vi "Autonomous Independent.vi"() -> ()   [LabVIEW 2015]
doc: "This VI is called when autonomous begins, and will automatically be terminated when autonomous ends. You can carry out timed or sensor driven robot movement independently without needing to return to the caller."
uses:
  <vilib>/Rock Robotics/WPI/RobotDrive/WPI_RobotDriveDevRef.ctl
  <vilib>/Rock Robotics/WPI/MotorControl/WPI_MotorControlDeviceRef.ctl
  <vilib>/Rock Robotics/WPI/MotorControl/WPI_MotorControlType.ctl
  <vilib>/Rock Robotics/SystemInterfaces/DIO/FPGA_DIOPWMChannel.ctl
  <vilib>/Rock Robotics/WPI/PWM/WPI_PWMDeadband.ctl
  <vilib>/Rock Robotics/WPI/CAN/Jaguar/SubVIs/WPI_CANJaguar_ControlMode.ctl
  <vilib>/Rock Robotics/WPI/CAN/TalonSRX/WPI_CANTalonSRX_APIControlMode.ctl
  <vilib>/Rock Robotics/WPI/Encoder/WPI_EncoderDevRef.ctl
  <vilib>/Rock Robotics/SystemInterfaces/Encoder/FPGA_EncoderIdx.ctl
  <vilib>/Rock Robotics/SystemInterfaces/Counter/FPGA_CounterCtrSystemIndex.ctl
  <vilib>/Rock Robotics/WPI/Encoder/WPI_EncoderType.ctl
  <vilib>/Rock Robotics/WPI/Utilities/WPI_GetSetVariantRefNum.vi
  Robot Global Data.vi
panel:
  in  "stop?":bool
  out "Pot Position":dbl
  in  "Angle(degrees)":dbl
  out "End?":bool
  out "End?":bool
  in  "Gear Setting":bool=TRUE
  in  "Distance (in)":dbl
  in  "Auto Choice":T1(ring)=enum."Low Bar"
  # "Be sure to right-click and choose Data Operations>>Make Current Value default if you want to save the array values with the VI"
  # "Move Forward at Dist. Test"
  # "Move Arms Down/Up Test"
  # "Low"
  # "High"
  # "<<Turn Until Vision Test"
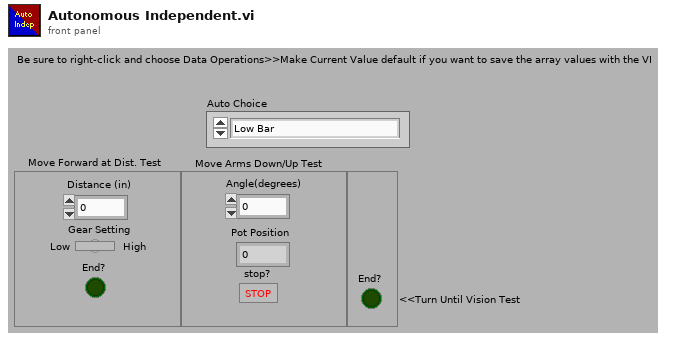
[diagram p1: front panel]
types:
  T1 = enum16{"Spybox/Shooting Test", "Low Bar", "Position 2", "Position 3", "Position 4", "Position 5", "Move Arms Down/Up Test", "Move Forward at Dist. Test", "Turn Until Vision Test"}
  T2 = typedef "WPI_RobotDriveDevRef.ctl" = cluster{"DevStatus":errorcluster, "Motors[]":T3[], "Square Inputs":bool, "Max Output":dbl}
  T3 = typedef "WPI_MotorControlDeviceRef.ctl" = cluster{"DeviceStatus":errorcluster, "Type":T4, "PWM":cluster{"PWM Channel":T5, "DeadBand":T6}, "CAN":cluster{"Device Number":u8, "Control Mode":T7, "Semaphore":T8, "Max Vout":dbl, "TalonSRX Control Mode":T9}, "Invert":bool}
  T4 = typedef "WPI_MotorControlType.ctl" = enum16{"PWM", "CAN", "CANTalonSRX"}
  T5 = typedef "FPGA_DIOPWMChannel.ctl" = enum8{"PWM 0", "PWM 1", "PWM 2", "PWM 3", "PWM 4", "PWM 5", "PWM 6", "PWM 7", "PWM 8", "PWM 9", "PWM MXP 0", "PWM MXP 1", "PWM MXP 2", "PWM MXP 3", "PWM MXP 4", "PWM MXP 5", "PWM MXP 6", "PWM MXP 7", "PWM MXP 8", "PWM MXP 9", "Invalid"}
  T6 = typedef "WPI_PWMDeadband.ctl" = cluster{"Name":string, "maxPositivePwm":i32, "minPositivePwm":i32, "centerPwm":i32, "maxNegativePwm":i32, "minNegativePwm":i32, "angularRange":u16}
  T7 = typedef "WPI_CANJaguar_ControlMode.ctl" = enum8{"Percent VBus", "Current", "Speed", "Position", "Voltage"}
  T8 = typedef "Semaphore RefNum" = refnum<k1>
  T9 = typedef "WPI_CANTalonSRX_APIControlMode.ctl" = enum8{"Percent VBus", "Speed", "Position", "Slave", "Unchanged / Invalid", "Voltage Compensation", "Current", "Motion Profile"}
  T10 = typedef "WPI_EncoderDevRef.ctl" = cluster{"DevStatus":errorcluster, "EncoderIndex":T11, "CounterIndex":T12, "DistancePerCount":dbl, "Decoding Type":T13}
  T11 = typedef "FPGA_EncoderIdx.ctl" = enum8{"Enc 0", "Enc 1", "Enc 2", "Enc 3", "Enc 4", "Enc 5", "Enc 6", "Enc 7", "Invalid"}
  T12 = typedef "FPGA_CounterCtrSystemIndex.ctl" = enum8{"Ctr 0", "Ctr 1", "Ctr 2", "Ctr 3", "Ctr 4", "Ctr 5", "Ctr 6", "Ctr 7", "Invalid"}
  T13 = typedef "WPI_EncoderType.ctl" = enum16{"1x", "2x", "4x"}
  T14 = cluster{"DriveRef":T2, "LeftEncRef":T10, "RightEncRef":T10}
  T15 = typedef "WPI_CANTalonSRX_GlobalStatus.ctl" = cluster{"Applied Throttle":dbl, "Module Enabled":bool, "CAN Error":errorcluster, "Closed Loop Error":dbl, "Forward Limit Switch Closed":bool, "Reverse Limit Switch Closed":bool, "Sensor Position":dbl, "Sensor Velocity":dbl, "Current":dbl, "Sticky Fault - Over Temp":bool, "Sticky Fault - Under Voltage":bool, "Sticky Fault - Forward Limit":bool, "Sticky Fault - Reverse Limit":bool, "Sticky Fault - Forward Soft Limit":bool, "Sticky Fault - Reverse Soft Limit":bool, "Brake is Enabled":bool, "Encoder Position":dbl, "Encoder Velocity":dbl, "Encoder Index Count":dbl, "Encoder A Pin State":bool, "Encoder B Pin State":bool, "Encoder Index Pin State":bool, "Analog In":dbl, "Analog In Velocity":dbl, "Temperature (C)":dbl, "Battery Voltage":dbl, "Control 5 Is Supported":bool, "Current Profile Slot Select":dbl, "Pos Div 8":bool, "Vel Div 4":bool, "Pulse Width Position":i32, "Pulse Width Velocity":i32, "Pulse Width Rise To Rise (us)":i32, "Pulse Width Rise To Fall (us)":i32, "Mot Prof Active Is Under Run":bool, "Mot Prof Active Has Under Run":bool, "Mot Prof Active Is Last":bool, "Mot Prof Active Velocity Only":bool, "Mot Prof Active Is Valid":bool, "Mot Prof Buffer Is Full":bool, "Mot Prof Active Profile Slot Select":i32, "Mot Prof NextID":i32, "Mot Prof Count":i32, "Mot Prof Active Velocity":dbl, "Mot Prof Active Position":dbl, "Mot Prof Output Enable":i32}
  T16 = enum16{"Start", "Turn (No Vision)", "Turn (Vision)", "Shoot", "Turn Back", "Move Back", "End"}
  T17 = cluster{"Angle":dbl, "Distance":dbl, "x":dbl, "y":dbl}
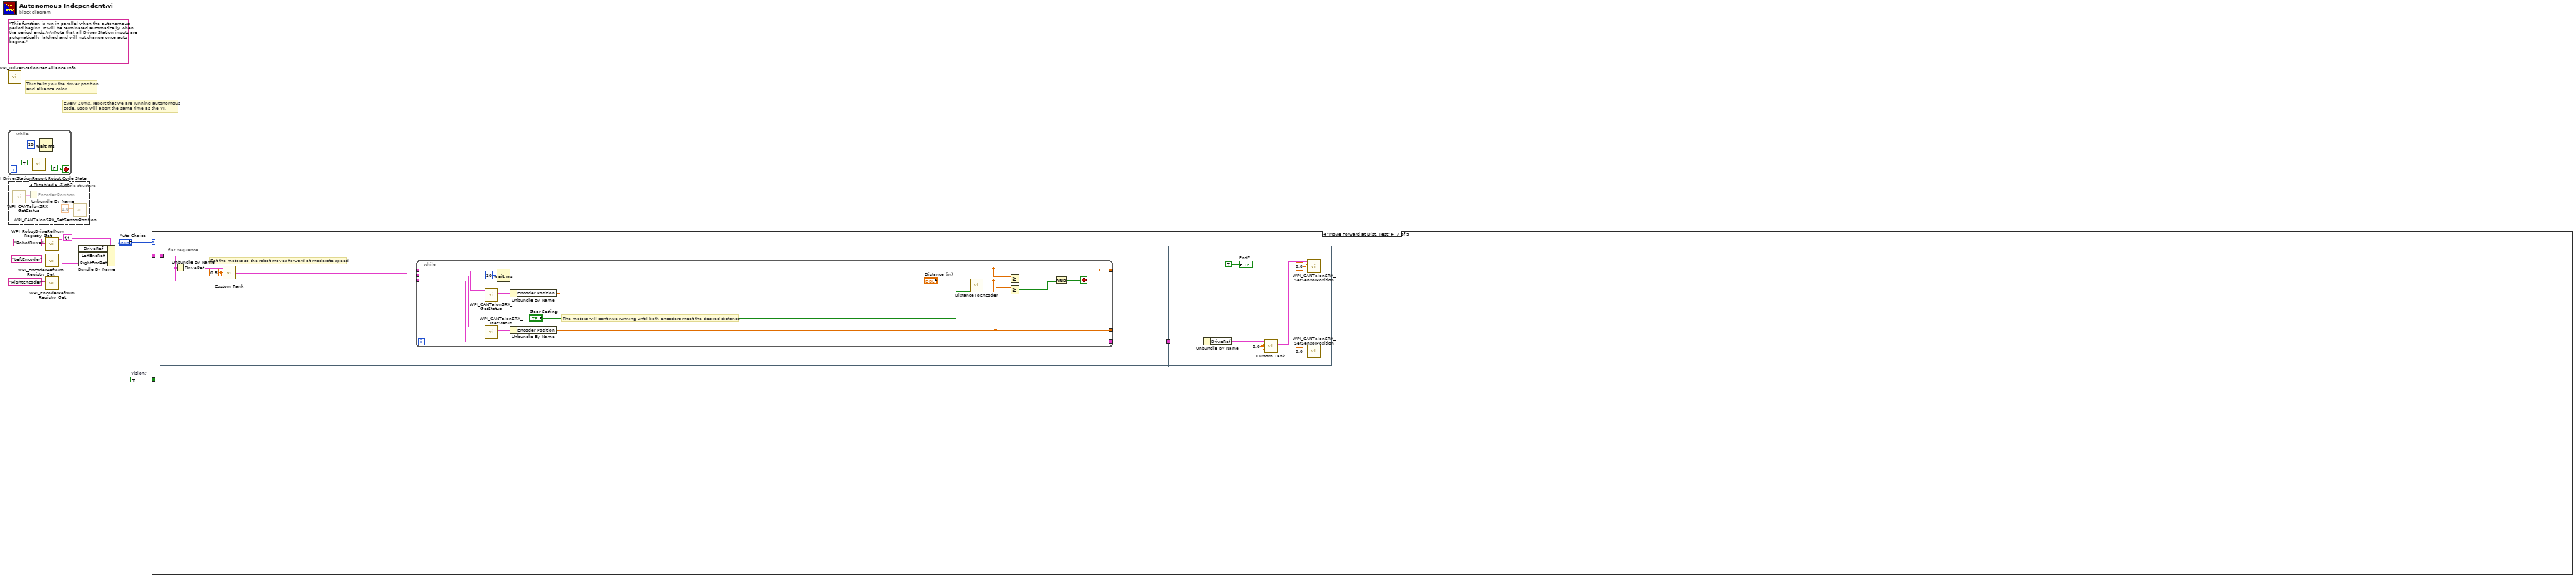
[diagram p0: block diagram]
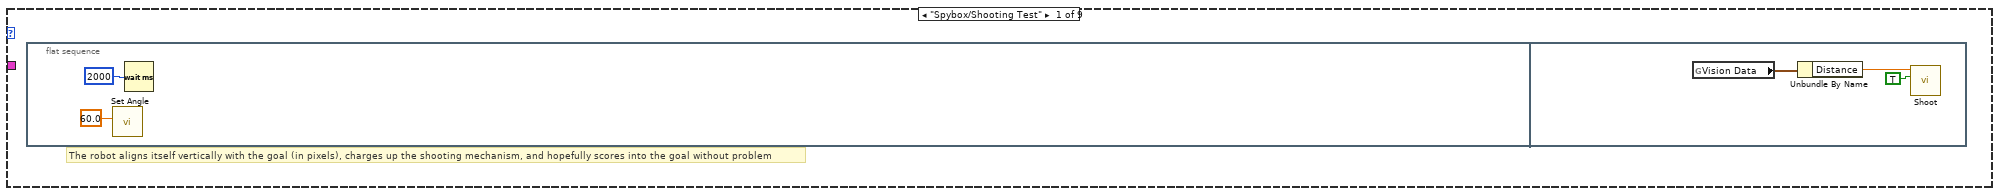
[diagram p3: hidden frame]
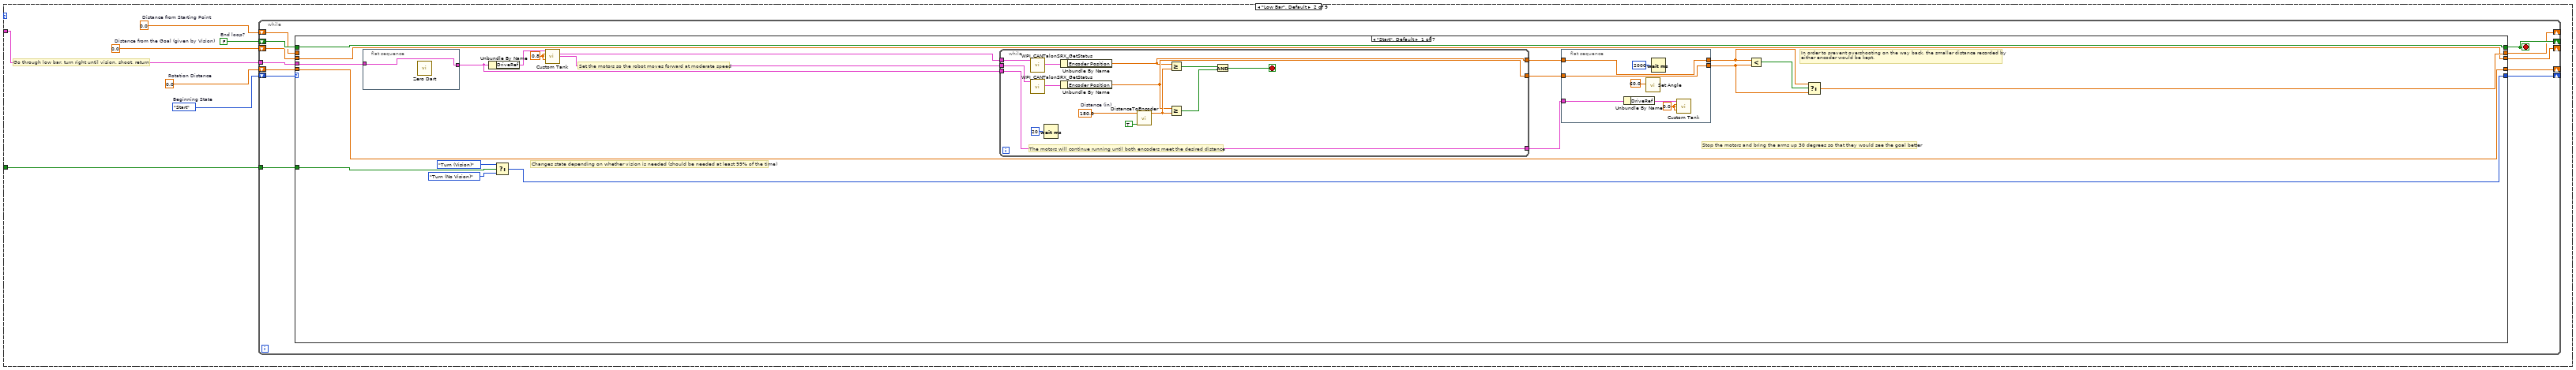
[diagram p4: hidden frame]
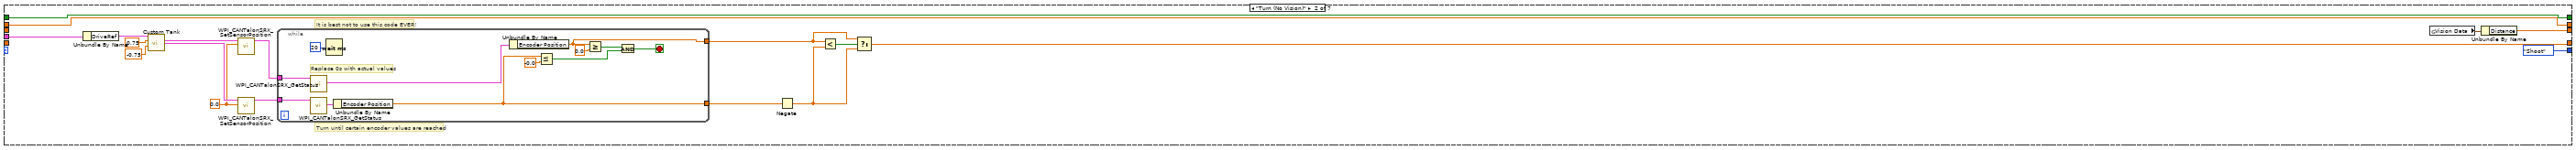
[diagram p5: hidden frame]
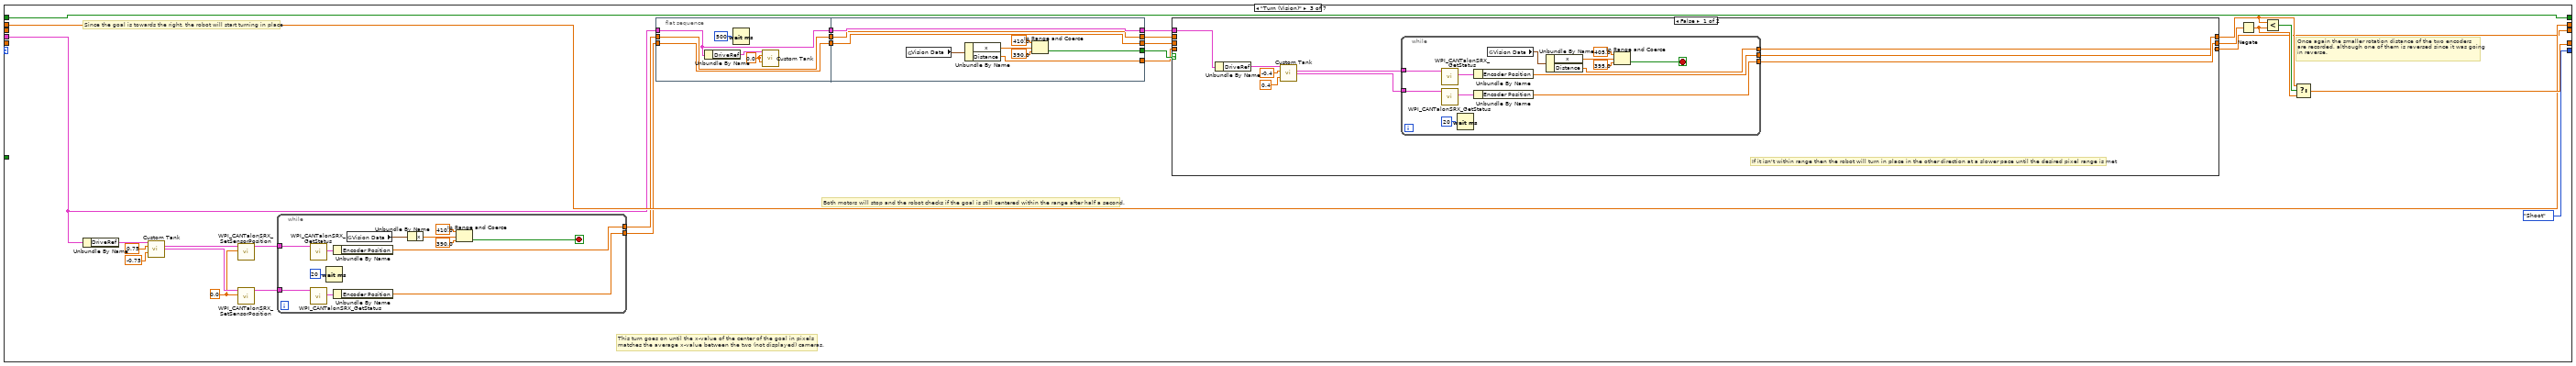
[diagram p6: hidden frame]
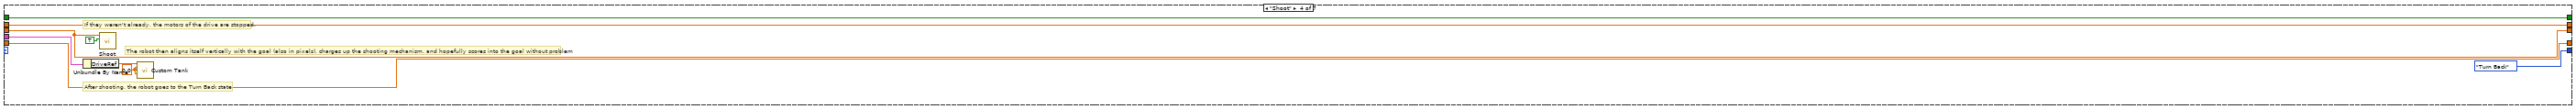
[diagram p8: hidden frame]
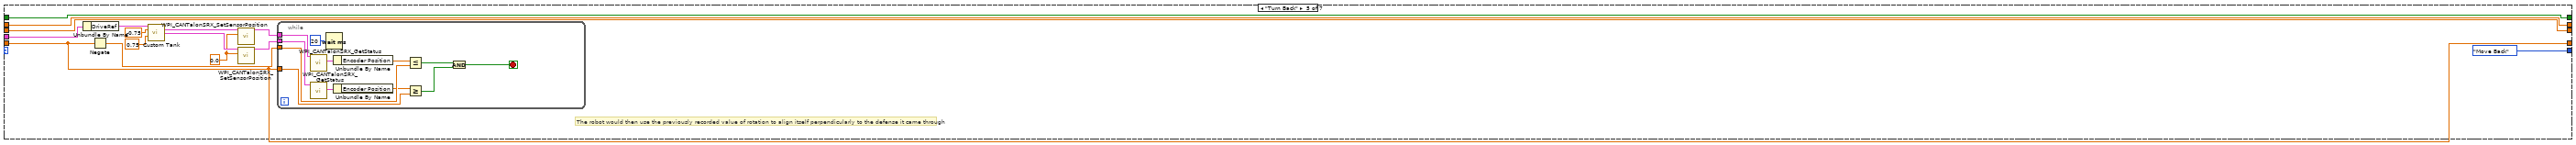
[diagram p9: hidden frame]
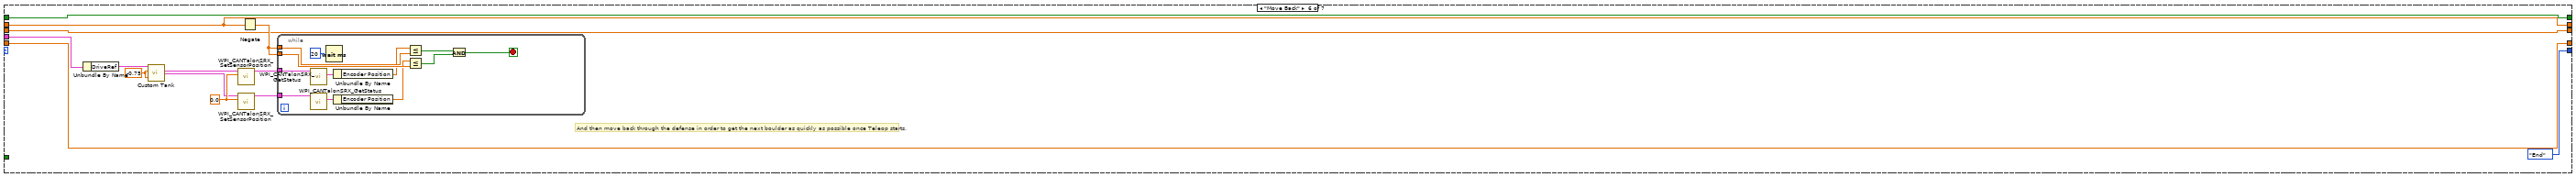
[diagram p10: hidden frame]
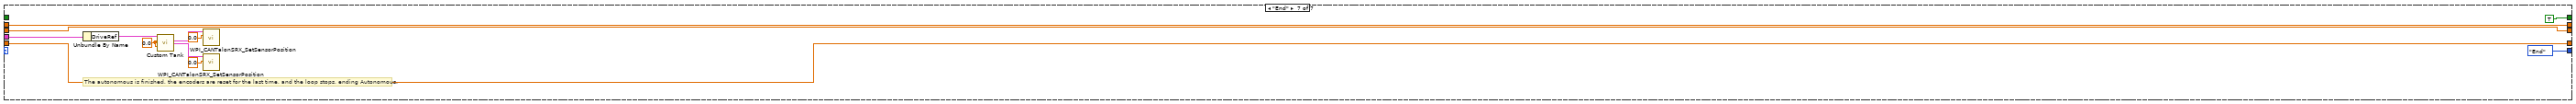
[diagram p11: hidden frame]
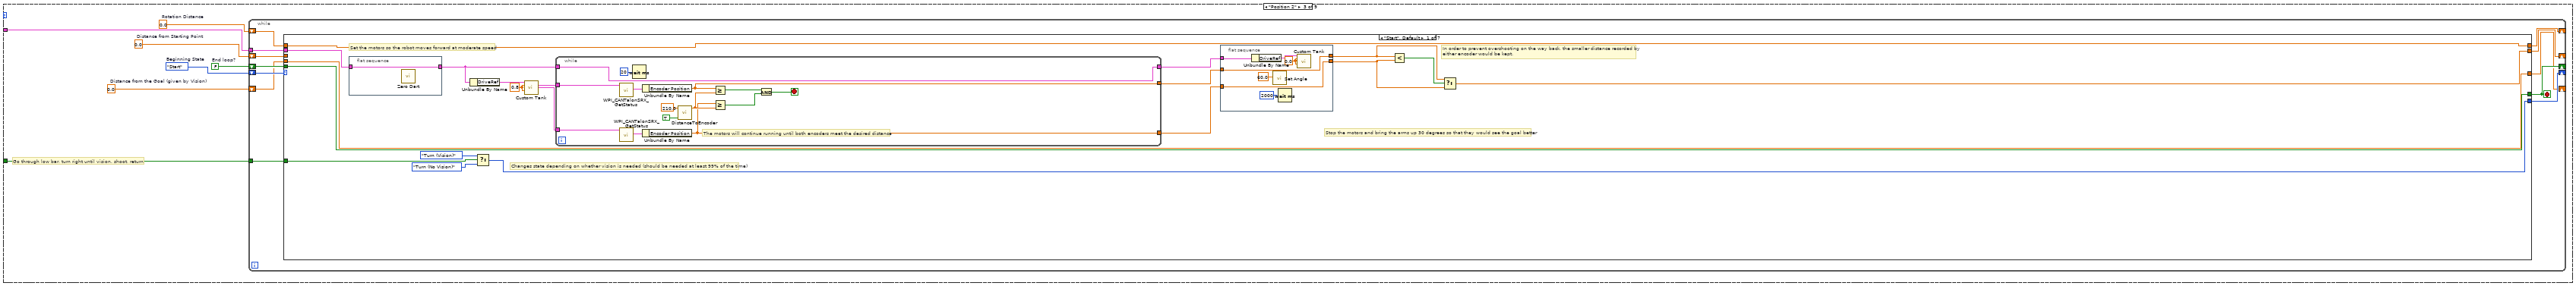
[diagram p12: hidden frame]
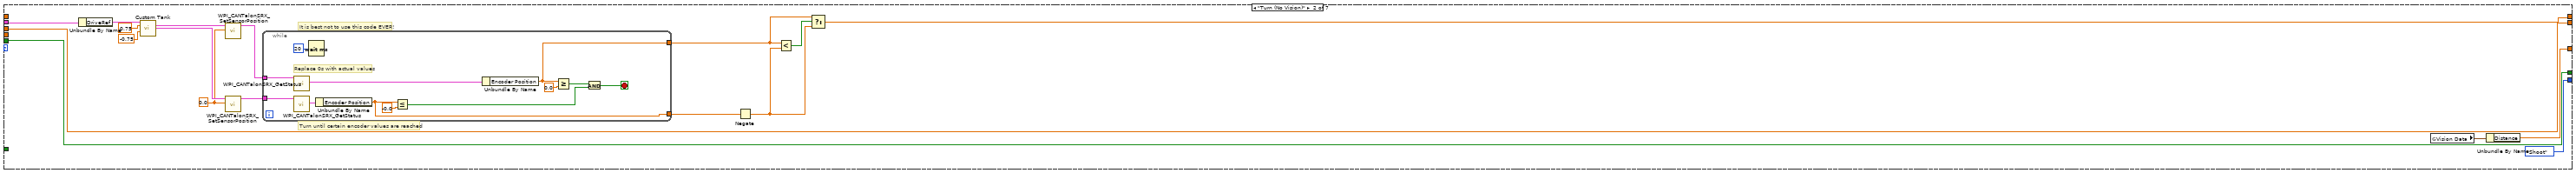
[diagram p13: hidden frame]
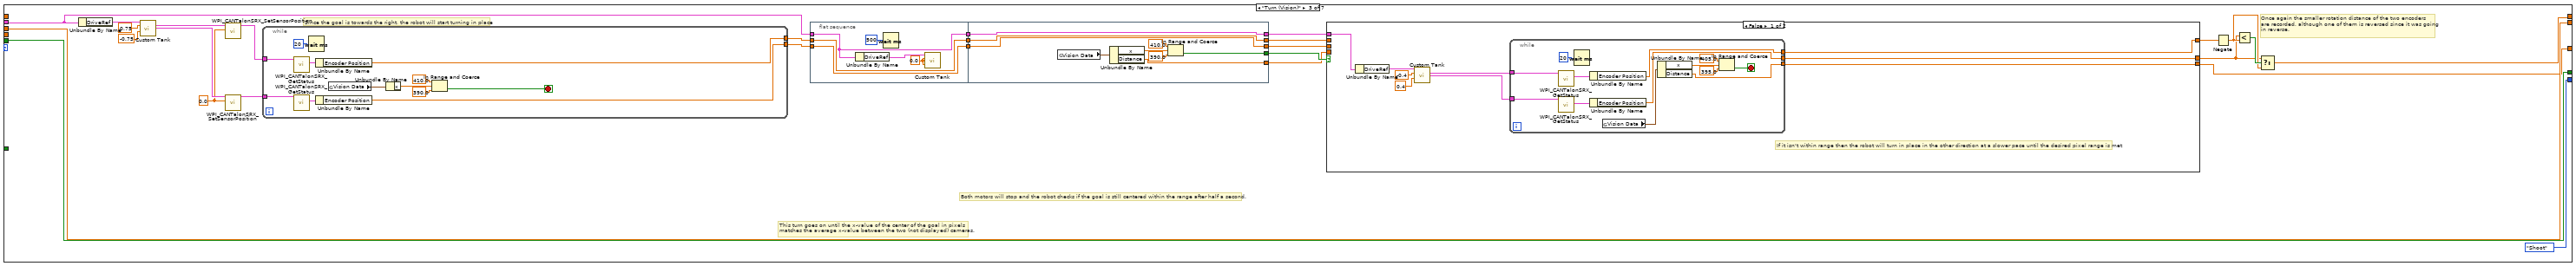
[diagram p14: hidden frame]
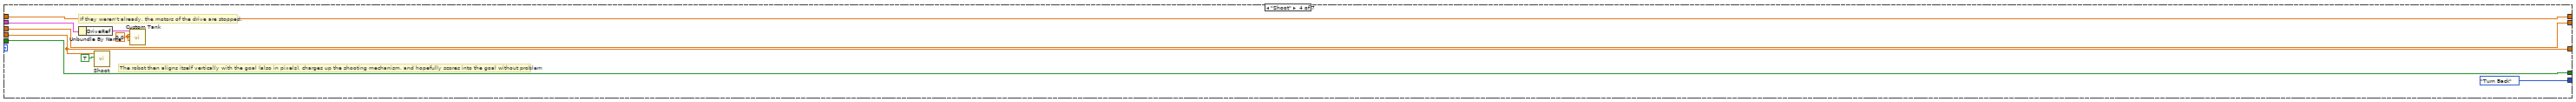
[diagram p16: hidden frame]
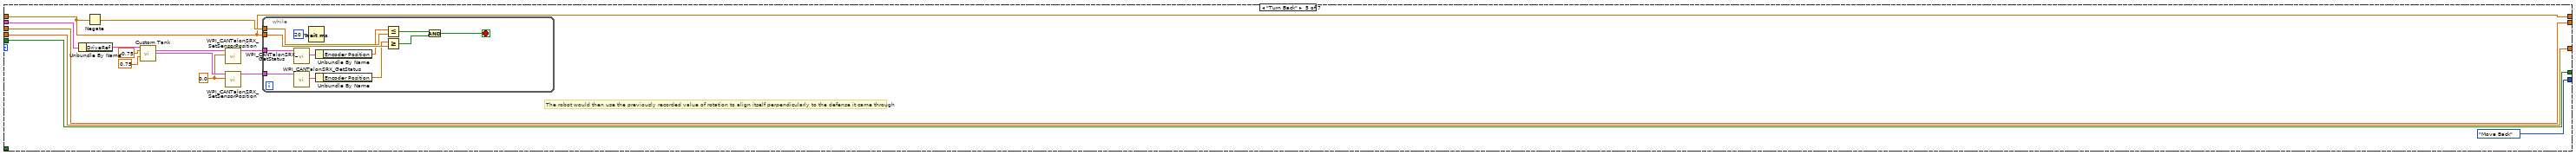
[diagram p17: hidden frame]
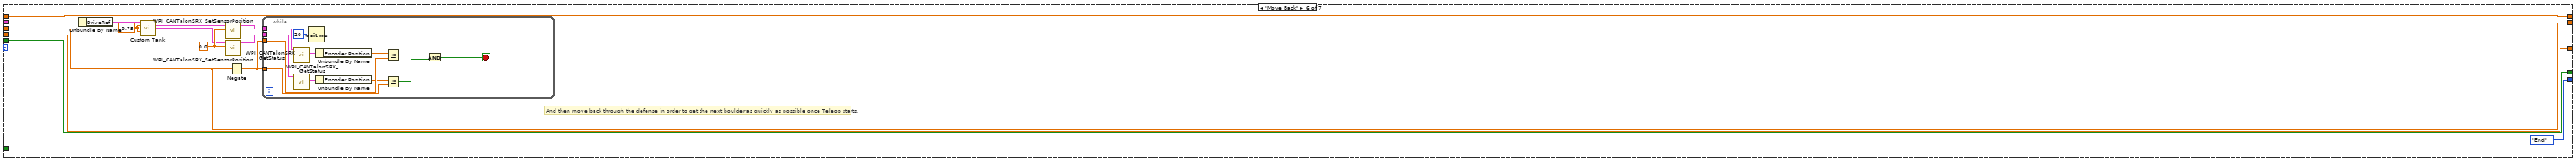
[diagram p18: hidden frame]
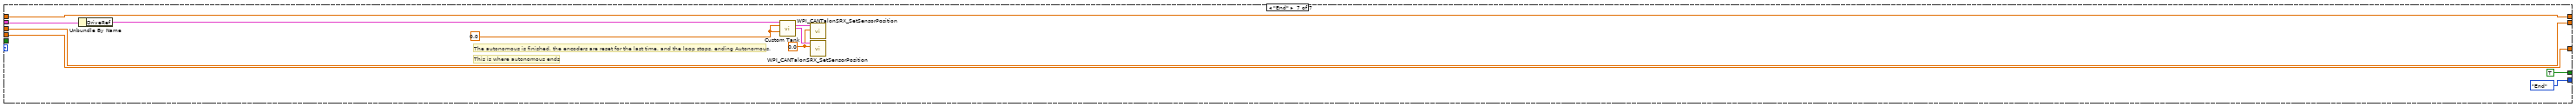
[diagram p19: hidden frame]
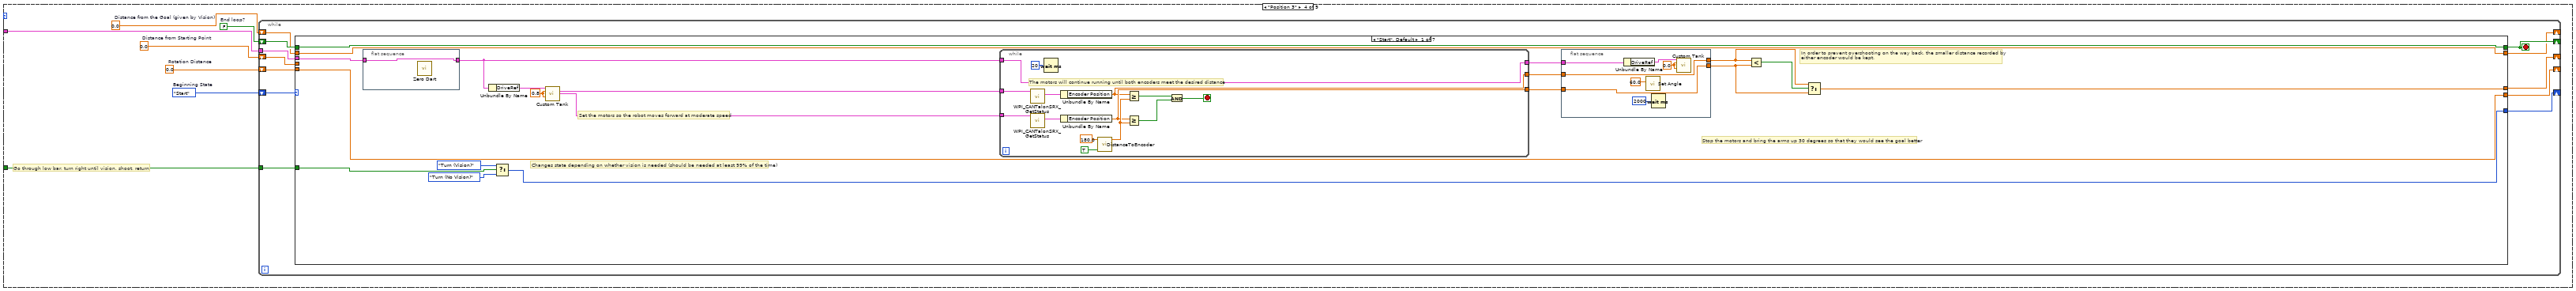
[diagram p20: hidden frame]
diagram:
  w10 = TRUE  # Vision?
  (unwired) "This function is run in parallel when the autonomous period begins. It will be terminated automatically when the period ends.\n\nNote that all Driver Station inputs are automatically latched and will not change once auto begins."
  # "Every 20ms, report that we are running autonomous\ncode. Loop will abort the same time as the VI."
  # "This tells you the driver position\nand alliance color"
  n1 = call <vilib>:"WPI_DriverStationGet Alliance Info.vi"() -> ()  [unwired: 12 out]
  n2 = while {
    stop <- FALSE stop-if-true
    n3 = call <vilib>:"WPI_DriverStationReport Robot Code State.vi"("Autonomous"=TRUE) -> ()  [unwired: 10 in, 1 out]
    n4 = Wait (ms)(milliseconds to wait=u32 20) -> ()  [unwired: 1 out]
  }
  n5 = disable-structure shown="Disabled" {
    frame Disabled {
      n6 = call <vilib>:"WPI_CANTalonSRX_GetStatus.vi"() -> ("Talon SRX Status"=w15:T15)  [unwired: 9 in, 2 out]
      n7 = Unbundle By Name(w15) -> ()  [unwired: 1 out]
      n8 = call <vilib>:"WPI_CANTalonSRX_SetSensorPosition.vi"("New Sensor Position"=0.0) -> ()  [unwired: 9 in, 2 out]
    }
    frame Enabled {
    }
  }
  n9 = call <vilib>:"WPI_RobotDriveRefNum Registry Get.vi"("refnum name"="RobotDrive") -> ("RobotDriveDevRef"=w5:T2)  [unwired: 9 in, 1 out]
  n10 = call <vilib>:"WPI_EncoderRefNum Registry Get.vi"("refnum name"="LeftEncoder") -> ("EncoderDevRef"=w4:T10)  [unwired: 9 in, 1 out]
  n11 = call <vilib>:"WPI_EncoderRefNum Registry Get.vi"("refnum name"="RightEncoder") -> ("EncoderDevRef"=w3:T10)  [unwired: 9 in, 1 out]
  n12 = Bundle By Name(cluster=T14 {"DriveRef"={"DevStatus"={"status"=FALSE, "code"=0, "source"=""}, "Motors[]"=[], "Square Inputs"=FALSE, "Max Output"=1.0}, "LeftEncRef"={"DevStatus"={"status"=FALSE, "code"=0, "source"=""}, "EncoderIndex"=enum."Invalid", "CounterIndex"=enum."Invalid", "DistancePerCount"=1.0, "Decoding Type"=enum."4x"}, "RightEncRef"={"DevStatus"={"status"=FALSE, "code"=0, "source"=""}, "EncoderIndex"=enum."Invalid", "CounterIndex"=enum."Invalid", "DistancePerCount"=1.0, "Decoding Type"=enum."4x"}}, "DriveRef"=w5, "LeftEncRef"=w4, "RightEncRef"=w3) -> (w2:T14)
  n13 = case shown="\"Move Forward at Dist. Test\"" "Auto Choice" {
    tunnel: w10 -> [_ w24 w268 w513 _ w869 _ _ _]
    tunnel: w2 -> [_ w21 w267 w512 w762 w868 w1120 w1151 _]
    frame "Spybox/Shooting Test" {
      # "The robot aligns itself vertically with the goal (in pixels), charges up the shooting mechanism, and hopefully scores into the goal without problem"
      n14 = flat-sequence {
        frame #0 {
          n15 = call "Set Angle.vi"("Angle(degrees)"=60.0) -> ()  [unwired: 7 in, 4 out]
          n16 = Wait (ms)(milliseconds to wait=u32 2000) -> ()  [unwired: 1 out]
        }
        frame #1 {
          n17 = global read "Robot Global Data.vi" "Vision Data"() -> (w18:T17)
          n18 = Unbundle By Name(w18) -> ("Distance"=w20:dbl)
          n19 = call "Shoot.vi"("Trigger"=TRUE ("Aimbot?"), "Vision Distance"=w20) -> ()  [unwired: 7 in, 3 out]
        }
      }
    }
    frame "Low Bar", Default {
      w27 = 0.0  # Distance from the Goal (given by Vision)
      w23 = 0.0  # Rotation Distance
      w22 = 0.0  # Distance from Starting Point
      w25 = FALSE  # End loop?
      w26 = T16."Start"  # Beginning State
      # "Go through low bar, turn right until vision, shoot, return"
      n20 = while {
        shift-right: [w39] -> _
        shift-left: w26 -> [w29]
        shift-right: [w37] -> _
        shift-left: w25 -> [w38]
        shift-right: [w35] -> _
        shift-left: w22 -> [w36]
        shift-right: [w33] -> _
        shift-left: w23 -> [w34]
        shift-right: [w31] -> _
        shift-left: w27 -> [w32]
        tunnel: w24 -> [w30]
        tunnel: w21 -> [w28]
        stop <- w37 stop-if-true
        n21 = case shown="\"Start\", Default" w29 {
          tunnel: [w59 T16."Shoot" T16."Shoot" T16."Turn Back" T16."Move Back" T16."End" T16."End"] -> w39
          tunnel: [w58 w99 w136 w201 w215 w241 TRUE] -> w37
          tunnel: w38 -> [w58 w99 w136 w201 w215 w241 _]
          tunnel: [w52 w98 w135 w196 w214 w238 w264] -> w35
          tunnel: w36 -> [_ w98 w135 w196 w214 w238 w264]
          tunnel: w34 -> [w51 _ _ w199 w212 w240 w263]
          tunnel: [w51 w93 w137 w199 w212 w240 w263] -> w33
          tunnel: w32 -> [w46 _ _ w195 w211 w237 w262]
          tunnel: [w46 w91 w122 w195 w211 w237 w262] -> w31
          tunnel: w30 -> [w50 _ _ _ _ _ _]
          tunnel: w28 -> [w45 w90 w134 w198 w210 w236 w261]
          frame "Start", Default {
            w42 = 0.8 ("LeftMotorsSpeed")
            # "In order to prevent overshooting on the way back, the smaller distance recorded by\neither encoder would be kept."
            # "Stop the motors and bring the arms up 30 degrees so that they would see the goal better"
            # "Set the motors so the robot moves forward at moderate speed"
            # "Changes state depending on whether vision is needed (should be needed at least 99% of the time)"
            n22 = flat-sequence {
              tunnel: w45 -> [w60]
              tunnel: [w60] -> w44
              frame #0 {
                n23 = call "Zero Dart.vi"() -> ()  [unwired: 10 in, 2 out]
              }
            }
            n24 = Unbundle By Name(w44) -> ("DriveRef"=w43:T2)
            n25 = Select(t=T16."Turn (Vision)", s=w50, f=T16."Turn (No Vision)") -> (s? t:f=w59:T16)
            n26 = call "Custom Tank.vi"("RobotDriveDevRef 2"=w43, "Left axis value"=w42, "Right axis value"=w42) -> ("Middle Left Motor"=w41:T3, "Middle Right Motor"=w40:T3)  [unwired: 8 in, 3 out]
            n27 = while {
              tunnel: [w61] -> w48
              tunnel: [w62] -> w47
              tunnel: w44 -> [w67]
              tunnel: [w67] -> w49
              tunnel: w41 -> [w64]
              tunnel: w40 -> [w63]
              stop <- w72 stop-if-true
              w70 = 180.0  # Distance (in)
              # "The motors will continue running until both encoders meet the desired distance"
              n28 = call <vilib>:"WPI_CANTalonSRX_GetStatus.vi"("CAN Talon SRX Ref"=w64) -> ("Talon SRX Status"=w66:T15)  [unwired: 8 in, 2 out]
              n29 = call <vilib>:"WPI_CANTalonSRX_GetStatus.vi"("CAN Talon SRX Ref"=w63) -> ("Talon SRX Status"=w65:T15)  [unwired: 8 in, 2 out]
              n30 = Wait (ms)(milliseconds to wait=u32 20) -> ()  [unwired: 1 out]
              n31 = Unbundle By Name(w66) -> ("Encoder Position"=w61:dbl)
              n32 = Unbundle By Name(w65) -> ("Encoder Position"=w62:dbl)
              n33 = call "DistanceToEncoder.vi"("Gear Setting"=TRUE, "Distance (in)"=w70) -> ("Encoder Ticks"=w69:dbl)  [unwired: 9 in]
              n34 = Greater Or Equal?(x=w61, y=w69) -> (x >= y?=w74:bool)
              n35 = Greater Or Equal?(x=w62, y=w69) -> (x >= y?=w73:bool)
              n36 = And(x=w74, y=w73) -> (x .and. y?=w72:bool)
            }
            n37 = flat-sequence {
              tunnel: [w78] -> w54
              tunnel: [w77] -> w53
              tunnel: w49 -> [w79]
              tunnel: w48 -> [w78]
              tunnel: w47 -> [w77]
              frame #0 {
                w75 = 0.0 ("LeftMotorsSpeed")
                n38 = Unbundle By Name(w79) -> ("DriveRef"=w76:T2)
                n39 = call "Set Angle.vi"("Angle(degrees)"=60.0) -> ()  [unwired: 7 in, 4 out]
                n40 = Wait (ms)(milliseconds to wait=u32 2000) -> ()  [unwired: 1 out]
                n41 = call "Custom Tank.vi"("RobotDriveDevRef 2"=w76, "Left axis value"=w75, "Right axis value"=w75) -> ()  [unwired: 8 in, 5 out]
              }
            }
            n42 = Less?(x=w54, y=w53) -> (x < y?=w55:bool)
            n43 = Select(t=w54, s=w55, f=w53) -> (s? t:f=w52:dbl)
          }
          frame "Turn (No Vision)" {
            w82 = 0.0 ("New Sensor Position")
            # "It is best not to use this code EVER!"
            # "Turn until certain encoder values are reached"
            n44 = Unbundle By Name(w90) -> ("DriveRef"=w89:T2)
            n45 = call "Custom Tank.vi"("RobotDriveDevRef 2"=w89, "Left axis value"=0.75 ("LeftMotorsSpeed"), "Right axis value"=-0.75 ("RightMotorsSpeed")) -> ("Middle Left Motor"=w86:T3, "Middle Right Motor"=w85:T3)  [unwired: 8 in, 3 out]
            n46 = call <vilib>:"WPI_CANTalonSRX_SetSensorPosition.vi"("New Sensor Position"=w82, "CAN Talon SRX Ref"=w86) -> ("CAN Talon SRX Ref"=w84:T3)  [unwired: 8 in, 1 out]
            n47 = call <vilib>:"WPI_CANTalonSRX_SetSensorPosition.vi"("New Sensor Position"=w82, "CAN Talon SRX Ref"=w85) -> ("CAN Talon SRX Ref"=w83:T3)  [unwired: 8 in, 1 out]
            n48 = while {
              tunnel: w84 -> [w105]
              tunnel: w83 -> [w103]
              tunnel: [w101] -> w95
              tunnel: [w102] -> w97
              stop <- w108 stop-if-true
              # "Replace 0s with actual values"
              n49 = call <vilib>:"WPI_CANTalonSRX_GetStatus.vi"("CAN Talon SRX Ref"=w105) -> ("Talon SRX Status"=w106:T15)  [unwired: 8 in, 2 out]
              n50 = call <vilib>:"WPI_CANTalonSRX_GetStatus.vi"("CAN Talon SRX Ref"=w103) -> ("Talon SRX Status"=w104:T15)  [unwired: 8 in, 2 out]
              n51 = Wait (ms)(milliseconds to wait=u32 20) -> ()  [unwired: 1 out]
              n52 = Unbundle By Name(w104) -> ("Encoder Position"=w102:dbl)
              n53 = Unbundle By Name(w106) -> ("Encoder Position"=w101:dbl)
              n54 = Less Or Equal?(x=w102, y=-0.0) -> (x <= y?=w110:bool)
              n55 = Greater Or Equal?(x=w101, y=0.0) -> (x >= y?=w111:bool)
              n56 = And(x=w111, y=w110) -> (x .and. y?=w108:bool)
            }
            n57 = Negate(x=w97) -> (-x=w94:dbl)
            n58 = Less?(x=w95, y=w94) -> (x < y?=w96:bool)
            n59 = Select(t=w95, s=w96, f=w94) -> (s? t:f=w93:dbl)
            n60 = global read "Robot Global Data.vi" "Vision Data"() -> (w92:T17)
            n61 = Unbundle By Name(w92) -> ("Distance"=w91:dbl)
          }
          frame "Turn (Vision)" {
            w113 = 0.0 ("New Sensor Position")
            # "This turn goes on until the x-value of the center of the goal in pixels\nmatches the average x-value between the two (not displayed) cameras."
            # "Once again the smaller rotation distance of the two encoders\nare recorded, although one of them is reversed since it was going\nin reverse."
            # "Both motors will stop and the robot checks if the goal is still centered within the range after half a second."
            # "Since the goal is towards the right, the robot will start turning in place"
            n62 = Unbundle By Name(w134) -> ("DriveRef"=w120:T2)
            n63 = call "Custom Tank.vi"("RobotDriveDevRef 2"=w120, "Left axis value"=0.75 ("LeftMotorsSpeed"), "Right axis value"=-0.75 ("RightMotorsSpeed")) -> ("Middle Left Motor"=w117:T3, "Middle Right Motor"=w116:T3)  [unwired: 8 in, 3 out]
            n64 = call <vilib>:"WPI_CANTalonSRX_SetSensorPosition.vi"("New Sensor Position"=w113, "CAN Talon SRX Ref"=w117) -> ("CAN Talon SRX Ref"=w115:T3)  [unwired: 8 in, 1 out]
            n65 = call <vilib>:"WPI_CANTalonSRX_SetSensorPosition.vi"("New Sensor Position"=w113, "CAN Talon SRX Ref"=w116) -> ("CAN Talon SRX Ref"=w114:T3)  [unwired: 8 in, 1 out]
            n66 = while {
              tunnel: [w169] -> w132
              tunnel: [w168] -> w133
              tunnel: w115 -> [w167]
              tunnel: w114 -> [w166]
              stop <- w173 stop-if-true
              n67 = call <vilib>:"WPI_CANTalonSRX_GetStatus.vi"("CAN Talon SRX Ref"=w167) -> ("Talon SRX Status"=w171:T15)  [unwired: 8 in, 2 out]
              n68 = call <vilib>:"WPI_CANTalonSRX_GetStatus.vi"("CAN Talon SRX Ref"=w166) -> ("Talon SRX Status"=w170:T15)  [unwired: 8 in, 2 out]
              n69 = Wait (ms)(milliseconds to wait=u32 20) -> ()  [unwired: 1 out]
              n70 = Unbundle By Name(w171) -> ("Encoder Position"=w168:dbl)
              n71 = Unbundle By Name(w170) -> ("Encoder Position"=w169:dbl)
              n72 = global read "Robot Global Data.vi" "Vision Data"() -> (w177:T17)
              n73 = Unbundle By Name(w177) -> ("x"=w176:dbl)
              n74 = In Range and Coerce(upper limit=410.0, x=w176, lower limit=390.0) -> (In Range?=w173:bool)  [unwired: 1 out]
            }
            n75 = flat-sequence {
              tunnel: w134 -> [w182]
              tunnel: w133 -> [w181]
              tunnel: w132 -> [w180]
              tunnel: [w182] -> w126
              tunnel: [w181] -> w125
              tunnel: [w180] -> w124
              tunnel: [w190] -> w127
              tunnel: [w191] -> w128
              tunnel: [w192] -> w129
              tunnel: w126 -> [w192]
              tunnel: w125 -> [w191]
              tunnel: w124 -> [w190]
              tunnel: [w185] -> w123
              tunnel: [w184] -> w121
              frame #0 {
                w178 = 0.0 ("LeftMotorsSpeed")
                n76 = Unbundle By Name(w182) -> ("DriveRef"=w179:T2)
                n77 = Wait (ms)(milliseconds to wait=u32 500) -> ()  [unwired: 1 out]
                n78 = call "Custom Tank.vi"("RobotDriveDevRef 2"=w179, "Left axis value"=w178, "Right axis value"=w178) -> ()  [unwired: 8 in, 5 out]
              }
              frame #1 {
                n79 = global read "Robot Global Data.vi" "Vision Data"() -> (w189:T17)
                n80 = Unbundle By Name(w189) -> ("x"=w188:dbl, "Distance"=w184:dbl)
                n81 = In Range and Coerce(upper limit=410.0, x=w188, lower limit=390.0) -> (In Range?=w185:bool)  [unwired: 1 out]
              }
            }
            n82 = case shown="False" w123 {
              tunnel: [w148 w165] -> w130
              tunnel: w127 -> [_ w165]
              tunnel: w128 -> [_ w164]
              tunnel: [w149 w164] -> w131
              tunnel: w129 -> [w147 _]
              tunnel: [w146 w163] -> w122
              tunnel: w121 -> [_ w163]
              frame False {
                # "If it isn't within range then the robot will turn in place in the other direction at a slower pace until the desired pixel range is met"
                n83 = Unbundle By Name(w147) -> ("DriveRef"=w145:T2)
                n84 = call "Custom Tank.vi"("RobotDriveDevRef 2"=w145, "Left axis value"=-0.4 ("LeftMotorsSpeed"), "Right axis value"=0.4 ("RightMotorsSpeed")) -> ("Middle Left Motor"=w141:T3, "Middle Right Motor"=w142:T3)  [unwired: 8 in, 3 out]
                n85 = while {
                  tunnel: [w153] -> w149
                  tunnel: [w152] -> w148
                  tunnel: [w156] -> w146
                  tunnel: w142 -> [w151]
                  tunnel: w141 -> [w150]
                  stop <- w162 stop-if-true
                  n86 = call <vilib>:"WPI_CANTalonSRX_GetStatus.vi"("CAN Talon SRX Ref"=w150) -> ("Talon SRX Status"=w155:T15)  [unwired: 8 in, 2 out]
                  n87 = call <vilib>:"WPI_CANTalonSRX_GetStatus.vi"("CAN Talon SRX Ref"=w151) -> ("Talon SRX Status"=w154:T15)  [unwired: 8 in, 2 out]
                  n88 = Wait (ms)(milliseconds to wait=u32 20) -> ()  [unwired: 1 out]
                  n89 = Unbundle By Name(w155) -> ("Encoder Position"=w153:dbl)
                  n90 = Unbundle By Name(w154) -> ("Encoder Position"=w152:dbl)
                  n91 = global read "Robot Global Data.vi" "Vision Data"() -> (w161:T17)
                  n92 = Unbundle By Name(w161) -> ("x"=w160:dbl, "Distance"=w156:dbl)
                  n93 = In Range and Coerce(upper limit=405.0, x=w160, lower limit=395.0) -> (In Range?=w162:bool)  [unwired: 1 out]
                }
              }
              frame True {
                # "If it is within range, then the robot moves on to the shooting state"
              }
            }
            n94 = Negate(x=w130) -> (-x=w139:dbl)
            n95 = Less?(x=w131, y=w139) -> (x < y?=w140:bool)
            n96 = Select(t=w131, s=w140, f=w139) -> (s? t:f=w137:dbl)
          }
          frame "Shoot" {
            w193 = 0.0 ("LeftMotorsSpeed")
            # "After shooting, the robot goes to the Turn Back state"
            # "If they weren't already, the motors of the drive are stopped."
            # "The robot then aligns itself vertically with the goal (also in pixels), charges up the shooting mechanism, and hopefully scores into the goal without problem"
            n97 = Unbundle By Name(w198) -> ("DriveRef"=w194:T2)
            n98 = call "Shoot.vi"("Trigger"=TRUE ("Collection Trigger"), "Vision Distance"=w195) -> ()  [unwired: 7 in, 3 out]
            n99 = call "Custom Tank.vi"("RobotDriveDevRef 2"=w194, "Left axis value"=w193, "Right axis value"=w193) -> ()  [unwired: 8 in, 5 out]
          }
          frame "Turn Back" {
            w202 = 0.0 ("New Sensor Position")
            # "The robot would then use the previously recorded value of rotation to align itself perpendicularly to the defense it came through"
            n100 = Unbundle By Name(w210) -> ("DriveRef"=w209:T2)
            n101 = Negate(x=w212) -> (-x=w213:dbl)
            n102 = call "Custom Tank.vi"("RobotDriveDevRef 2"=w209, "Left axis value"=-0.75 ("LeftMotorsSpeed"), "Right axis value"=0.75 ("RightMotorsSpeed")) -> ("Middle Left Motor"=w203:T3, "Middle Right Motor"=w204:T3)  [unwired: 8 in, 3 out]
            n103 = call <vilib>:"WPI_CANTalonSRX_SetSensorPosition.vi"("New Sensor Position"=w202, "CAN Talon SRX Ref"=w203) -> ("CAN Talon SRX Ref"=w206:T3)  [unwired: 8 in, 1 out]
            n104 = call <vilib>:"WPI_CANTalonSRX_SetSensorPosition.vi"("New Sensor Position"=w202, "CAN Talon SRX Ref"=w204) -> ("CAN Talon SRX Ref"=w205:T3)  [unwired: 8 in, 1 out]
            n105 = while {
              tunnel: w206 -> [w218]
              tunnel: w205 -> [w217]
              tunnel: w212 -> [w225]
              tunnel: w213 -> [w224]
              stop <- w226 stop-if-true
              n106 = call <vilib>:"WPI_CANTalonSRX_GetStatus.vi"("CAN Talon SRX Ref"=w218) -> ("Talon SRX Status"=w222:T15)  [unwired: 8 in, 2 out]
              n107 = call <vilib>:"WPI_CANTalonSRX_GetStatus.vi"("CAN Talon SRX Ref"=w217) -> ("Talon SRX Status"=w221:T15)  [unwired: 8 in, 2 out]
              n108 = Wait (ms)(milliseconds to wait=u32 20) -> ()  [unwired: 1 out]
              n109 = Unbundle By Name(w222) -> ("Encoder Position"=w219:dbl)
              n110 = Unbundle By Name(w221) -> ("Encoder Position"=w220:dbl)
              n111 = Less Or Equal?(x=w219, y=w224) -> (x <= y?=w228:bool)
              n112 = Greater Or Equal?(x=w220, y=w225) -> (x >= y?=w227:bool)
              n113 = And(x=w228, y=w227) -> (x .and. y?=w226:bool)
            }
          }
          frame "Move Back" {
            w233 = 0.0 ("New Sensor Position")
            w234 = -0.75 ("LeftMotorsSpeed")
            # "And then move back through the defense in order to get the next boulder as quickly as possible once Teleop starts."
            n114 = Unbundle By Name(w236) -> ("DriveRef"=w235:T2)
            n115 = call "Custom Tank.vi"("RobotDriveDevRef 2"=w235, "Left axis value"=w234, "Right axis value"=w234) -> ("Middle Left Motor"=w232:T3, "Middle Right Motor"=w231:T3)  [unwired: 8 in, 3 out]
            n116 = call <vilib>:"WPI_CANTalonSRX_SetSensorPosition.vi"("New Sensor Position"=w233, "CAN Talon SRX Ref"=w232) -> ("CAN Talon SRX Ref"=w230:T3)  [unwired: 8 in, 1 out]
            n117 = call <vilib>:"WPI_CANTalonSRX_SetSensorPosition.vi"("New Sensor Position"=w233, "CAN Talon SRX Ref"=w231) -> ("CAN Talon SRX Ref"=w229:T3)  [unwired: 8 in, 1 out]
            n118 = Negate(x=w238) -> (-x=w239:dbl)
            n119 = while {
              tunnel: w230 -> [w246]
              tunnel: w229 -> [w243]
              tunnel: w239 -> [w251]
              tunnel: w239 -> [w250]
              stop <- w252 stop-if-true
              n120 = call <vilib>:"WPI_CANTalonSRX_GetStatus.vi"("CAN Talon SRX Ref"=w246) -> ("Talon SRX Status"=w248:T15)  [unwired: 8 in, 2 out]
              n121 = call <vilib>:"WPI_CANTalonSRX_GetStatus.vi"("CAN Talon SRX Ref"=w243) -> ("Talon SRX Status"=w245:T15)  [unwired: 8 in, 2 out]
              n122 = Wait (ms)(milliseconds to wait=u32 20) -> ()  [unwired: 1 out]
              n123 = Unbundle By Name(w248) -> ("Encoder Position"=w247:dbl)
              n124 = Unbundle By Name(w245) -> ("Encoder Position"=w244:dbl)
              n125 = Less Or Equal?(x=w247, y=w251) -> (x <= y?=w254:bool)
              n126 = Less Or Equal?(x=w244, y=w250) -> (x <= y?=w253:bool)
              n127 = And(x=w254, y=w253) -> (x .and. y?=w252:bool)
            }
          }
          frame "End" {
            w259 = 0.0 ("Left axis value")
            # "The autonomous is finished, the encoders are reset for the last time, and the loop stops, ending Autonomous."
            n128 = Unbundle By Name(w261) -> ("DriveRef"=w260:T2)
            n129 = call "Custom Tank.vi"("RobotDriveDevRef 2"=w260, "Left axis value"=w259, "Right axis value"=w259) -> ("Middle Left Motor"=w256:T3, "Middle Right Motor"=w255:T3)  [unwired: 8 in, 3 out]
            n130 = call <vilib>:"WPI_CANTalonSRX_SetSensorPosition.vi"("New Sensor Position"=0.0, "CAN Talon SRX Ref"=w256) -> ()  [unwired: 8 in, 2 out]
            n131 = call <vilib>:"WPI_CANTalonSRX_SetSensorPosition.vi"("New Sensor Position"=0.0, "CAN Talon SRX Ref"=w255) -> ()  [unwired: 8 in, 2 out]
          }
        }
      }
    }
    frame "Position 2" {
      w269 = 0.0  # Distance from the Goal (given by Vision)
      w270 = 0.0  # Rotation Distance
      w271 = 0.0  # Distance from Starting Point
      w272 = FALSE  # End loop?
      w273 = T16."Start"  # Beginning State
      # "Go through low bar, turn right until vision, shoot, return"
      n132 = while {
        shift-right: [w284] -> _
        shift-left: w273 -> [w285]
        shift-right: [w282] -> _
        shift-left: w272 -> [w283]
        shift-right: [w280] -> _
        shift-left: w271 -> [w281]
        shift-right: [w278] -> _
        shift-left: w270 -> [w279]
        shift-right: [w276] -> _
        shift-left: w269 -> [w277]
        tunnel: w268 -> [w275]
        tunnel: w267 -> [w274]
        stop <- w282 stop-if-true
        n133 = case shown="\"Start\", Default" w285 {
          tunnel: [w305 T16."Shoot" T16."Shoot" T16."Turn Back" T16."Move Back" T16."End" T16."End"] -> w284
          tunnel: [w304 w345 w382 w447 w456 w487 TRUE] -> w282
          tunnel: w283 -> [w304 w345 w382 w447 w456 w487 _]
          tunnel: [w298 w344 w381 w445 w461 w484 w509] -> w280
          tunnel: w281 -> [_ w344 w381 w445 w461 w484 w509]
          tunnel: w279 -> [w297 _ _ w444 w459 w486 w508]
          tunnel: [w297 w339 w383 w444 w459 w486 w508] -> w278
          tunnel: w277 -> [w296 _ _ w441 w458 w483 w507]
          tunnel: [w296 w337 w368 w441 w458 w483 w507] -> w276
          tunnel: w275 -> [w295 _ _ _ _ _ _]
          tunnel: w274 -> [w288 w336 w378 w443 w457 w482 w506]
          frame "Start", Default {
            w290 = 0.8 ("LeftMotorsSpeed")
            # "In order to prevent overshooting on the way back, the smaller distance recorded by\neither encoder would be kept."
            # "Stop the motors and bring the arms up 30 degrees so that they would see the goal better"
            # "Set the motors so the robot moves forward at moderate speed"
            # "Changes state depending on whether vision is needed (should be needed at least 99% of the time)"
            n134 = flat-sequence {
              tunnel: w288 -> [w306]
              tunnel: [w306] -> w289
              frame #0 {
                n135 = call "Zero Dart.vi"() -> ()  [unwired: 10 in, 2 out]
              }
            }
            n136 = Unbundle By Name(w289) -> ("DriveRef"=w291:T2)
            n137 = Select(t=T16."Turn (Vision)", s=w295, f=T16."Turn (No Vision)") -> (s? t:f=w305:T16)
            n138 = call "Custom Tank.vi"("RobotDriveDevRef 2"=w291, "Left axis value"=w290, "Right axis value"=w290) -> ("Middle Left Motor"=w287:T3, "Middle Right Motor"=w286:T3)  [unwired: 8 in, 3 out]
            n139 = while {
              tunnel: [w311] -> w293
              tunnel: [w309] -> w292
              tunnel: w289 -> [w313]
              tunnel: [w313] -> w294
              tunnel: w287 -> [w308]
              tunnel: w286 -> [w307]
              stop <- w318 stop-if-true
              # "The motors will continue running until both encoders meet the desired distance"
              n140 = call <vilib>:"WPI_CANTalonSRX_GetStatus.vi"("CAN Talon SRX Ref"=w308) -> ("Talon SRX Status"=w312:T15)  [unwired: 8 in, 2 out]
              n141 = call <vilib>:"WPI_CANTalonSRX_GetStatus.vi"("CAN Talon SRX Ref"=w307) -> ("Talon SRX Status"=w310:T15)  [unwired: 8 in, 2 out]
              n142 = Wait (ms)(milliseconds to wait=u32 20) -> ()  [unwired: 1 out]
              n143 = Unbundle By Name(w312) -> ("Encoder Position"=w311:dbl)
              n144 = Unbundle By Name(w310) -> ("Encoder Position"=w309:dbl)
              n145 = call "DistanceToEncoder.vi"("Gear Setting"=TRUE, "Distance (in)"=210.0 ("Distance")) -> ("Encoder Ticks"=w316:dbl)  [unwired: 9 in]
              n146 = Greater Or Equal?(x=w311, y=w316) -> (x >= y?=w320:bool)
              n147 = Greater Or Equal?(x=w309, y=w316) -> (x >= y?=w319:bool)
              n148 = And(x=w320, y=w319) -> (x .and. y?=w318:bool)
            }
            n149 = flat-sequence {
              tunnel: [w324] -> w300
              tunnel: [w323] -> w299
              tunnel: w294 -> [w325]
              tunnel: w293 -> [w324]
              tunnel: w292 -> [w323]
              frame #0 {
                w321 = 0.0 ("LeftMotorsSpeed")
                n150 = Unbundle By Name(w325) -> ("DriveRef"=w322:T2)
                n151 = call "Set Angle.vi"("Angle(degrees)"=60.0) -> ()  [unwired: 7 in, 4 out]
                n152 = Wait (ms)(milliseconds to wait=u32 2000) -> ()  [unwired: 1 out]
                n153 = call "Custom Tank.vi"("RobotDriveDevRef 2"=w322, "Left axis value"=w321, "Right axis value"=w321) -> ()  [unwired: 8 in, 5 out]
              }
            }
            n154 = Less?(x=w300, y=w299) -> (x < y?=w301:bool)
            n155 = Select(t=w300, s=w301, f=w299) -> (s? t:f=w298:dbl)
          }
          frame "Turn (No Vision)" {
            w330 = 0.0 ("New Sensor Position")
            # "It is best not to use this code EVER!"
            # "Turn until certain encoder values are reached"
            n156 = Unbundle By Name(w336) -> ("DriveRef"=w335:T2)
            n157 = call "Custom Tank.vi"("RobotDriveDevRef 2"=w335, "Left axis value"=0.75 ("LeftMotorsSpeed"), "Right axis value"=-0.75 ("RightMotorsSpeed")) -> ("Middle Left Motor"=w332:T3, "Middle Right Motor"=w331:T3)  [unwired: 8 in, 3 out]
            n158 = call <vilib>:"WPI_CANTalonSRX_SetSensorPosition.vi"("New Sensor Position"=w330, "CAN Talon SRX Ref"=w332) -> ("CAN Talon SRX Ref"=w329:T3)  [unwired: 8 in, 1 out]
            n159 = call <vilib>:"WPI_CANTalonSRX_SetSensorPosition.vi"("New Sensor Position"=w330, "CAN Talon SRX Ref"=w331) -> ("CAN Talon SRX Ref"=w328:T3)  [unwired: 8 in, 1 out]
            n160 = while {
              tunnel: w329 -> [w352]
              tunnel: w328 -> [w349]
              tunnel: [w350] -> w341
              tunnel: [w347] -> w343
              stop <- w354 stop-if-true
              # "Replace 0s with actual values"
              n161 = call <vilib>:"WPI_CANTalonSRX_GetStatus.vi"("CAN Talon SRX Ref"=w352) -> ("Talon SRX Status"=w351:T15)  [unwired: 8 in, 2 out]
              n162 = call <vilib>:"WPI_CANTalonSRX_GetStatus.vi"("CAN Talon SRX Ref"=w349) -> ("Talon SRX Status"=w348:T15)  [unwired: 8 in, 2 out]
              n163 = Wait (ms)(milliseconds to wait=u32 20) -> ()  [unwired: 1 out]
              n164 = Unbundle By Name(w348) -> ("Encoder Position"=w347:dbl)
              n165 = Less Or Equal?(x=w347, y=-0.0) -> (x <= y?=w356:bool)
              n166 = Unbundle By Name(w351) -> ("Encoder Position"=w350:dbl)
              n167 = Greater Or Equal?(x=w350, y=0.0) -> (x >= y?=w357:bool)
              n168 = And(x=w357, y=w356) -> (x .and. y?=w354:bool)
            }
            n169 = Negate(x=w343) -> (-x=w340:dbl)
            n170 = Less?(x=w341, y=w340) -> (x < y?=w342:bool)
            n171 = Select(t=w341, s=w342, f=w340) -> (s? t:f=w339:dbl)
            n172 = global read "Robot Global Data.vi" "Vision Data"() -> (w338:T17)
            n173 = Unbundle By Name(w338) -> ("Distance"=w337:dbl)
          }
          frame "Turn (Vision)" {
            w361 = 0.0 ("New Sensor Position")
            # "This turn goes on until the x-value of the center of the goal in pixels\nmatches the average x-value between the two (not displayed) cameras."
            # "Once again the smaller rotation distance of the two encoders\nare recorded, although one of them is reversed since it was going\nin reverse."
            # "Both motors will stop and the robot checks if the goal is still centered within the range after half a second."
            # "Since the goal is towards the right, the robot will start turning in place"
            n174 = Unbundle By Name(w378) -> ("DriveRef"=w366:T2)
            n175 = call "Custom Tank.vi"("RobotDriveDevRef 2"=w366, "Left axis value"=0.75 ("LeftMotorsSpeed"), "Right axis value"=-0.75 ("RightMotorsSpeed")) -> ("Middle Left Motor"=w363:T3, "Middle Right Motor"=w362:T3)  [unwired: 8 in, 3 out]
            n176 = call <vilib>:"WPI_CANTalonSRX_SetSensorPosition.vi"("New Sensor Position"=w361, "CAN Talon SRX Ref"=w363) -> ("CAN Talon SRX Ref"=w360:T3)  [unwired: 8 in, 1 out]
            n177 = call <vilib>:"WPI_CANTalonSRX_SetSensorPosition.vi"("New Sensor Position"=w361, "CAN Talon SRX Ref"=w362) -> ("CAN Talon SRX Ref"=w359:T3)  [unwired: 8 in, 1 out]
            n178 = while {
              tunnel: w360 -> [w416]
              tunnel: w359 -> [w413]
              tunnel: [w415] -> w380
              tunnel: [w412] -> w379
              stop <- w419 stop-if-true
              n179 = call <vilib>:"WPI_CANTalonSRX_GetStatus.vi"("CAN Talon SRX Ref"=w416) -> ("Talon SRX Status"=w417:T15)  [unwired: 8 in, 2 out]
              n180 = call <vilib>:"WPI_CANTalonSRX_GetStatus.vi"("CAN Talon SRX Ref"=w413) -> ("Talon SRX Status"=w414:T15)  [unwired: 8 in, 2 out]
              n181 = Wait (ms)(milliseconds to wait=u32 20) -> ()  [unwired: 1 out]
              n182 = Unbundle By Name(w417) -> ("Encoder Position"=w415:dbl)
              n183 = Unbundle By Name(w414) -> ("Encoder Position"=w412:dbl)
              n184 = global read "Robot Global Data.vi" "Vision Data"() -> (w423:T17)
              n185 = Unbundle By Name(w423) -> ("x"=w422:dbl)
              n186 = In Range and Coerce(upper limit=410.0, x=w422, lower limit=390.0) -> (In Range?=w419:bool)  [unwired: 1 out]
            }
            n187 = flat-sequence {
              tunnel: w380 -> [w426]
              tunnel: w379 -> [w427]
              tunnel: w378 -> [w428]
              tunnel: [w428] -> w372
              tunnel: [w427] -> w371
              tunnel: [w426] -> w370
              tunnel: [w436] -> w375
              tunnel: [w437] -> w376
              tunnel: [w438] -> w377
              tunnel: w372 -> [w438]
              tunnel: w371 -> [w437]
              tunnel: w370 -> [w436]
              tunnel: [w431] -> w369
              tunnel: [w430] -> w367
              frame #0 {
                w425 = 0.0 ("LeftMotorsSpeed")
                n188 = Unbundle By Name(w428) -> ("DriveRef"=w424:T2)
                n189 = Wait (ms)(milliseconds to wait=u32 500) -> ()  [unwired: 1 out]
                n190 = call "Custom Tank.vi"("RobotDriveDevRef 2"=w424, "Left axis value"=w425, "Right axis value"=w425) -> ()  [unwired: 8 in, 5 out]
              }
              frame #1 {
                n191 = global read "Robot Global Data.vi" "Vision Data"() -> (w435:T17)
                n192 = Unbundle By Name(w435) -> ("x"=w434:dbl, "Distance"=w430:dbl)
                n193 = In Range and Coerce(upper limit=410.0, x=w434, lower limit=390.0) -> (In Range?=w431:bool)  [unwired: 1 out]
              }
            }
            n194 = case shown="False" w369 {
              tunnel: [w394 w411] -> w374
              tunnel: w375 -> [_ w411]
              tunnel: w376 -> [_ w410]
              tunnel: [w395 w410] -> w373
              tunnel: w377 -> [w393 _]
              tunnel: [w392 w409] -> w368
              tunnel: w367 -> [_ w409]
              frame False {
                # "If it isn't within range then the robot will turn in place in the other direction at a slower pace until the desired pixel range is met"
                n195 = Unbundle By Name(w393) -> ("DriveRef"=w391:T2)
                n196 = call "Custom Tank.vi"("RobotDriveDevRef 2"=w391, "Left axis value"=-0.4 ("LeftMotorsSpeed"), "Right axis value"=0.4 ("RightMotorsSpeed")) -> ("Middle Left Motor"=w388:T3, "Middle Right Motor"=w387:T3)  [unwired: 8 in, 3 out]
                n197 = while {
                  tunnel: [w398] -> w395
                  tunnel: [w400] -> w394
                  tunnel: [w402] -> w392
                  tunnel: w388 -> [w397]
                  tunnel: w387 -> [w396]
                  stop <- w408 stop-if-true
                  n198 = call <vilib>:"WPI_CANTalonSRX_GetStatus.vi"("CAN Talon SRX Ref"=w397) -> ("Talon SRX Status"=w401:T15)  [unwired: 8 in, 2 out]
                  n199 = call <vilib>:"WPI_CANTalonSRX_GetStatus.vi"("CAN Talon SRX Ref"=w396) -> ("Talon SRX Status"=w399:T15)  [unwired: 8 in, 2 out]
                  n200 = Wait (ms)(milliseconds to wait=u32 20) -> ()  [unwired: 1 out]
                  n201 = Unbundle By Name(w401) -> ("Encoder Position"=w400:dbl)
                  n202 = Unbundle By Name(w399) -> ("Encoder Position"=w398:dbl)
                  n203 = global read "Robot Global Data.vi" "Vision Data"() -> (w407:T17)
                  n204 = Unbundle By Name(w407) -> ("x"=w406:dbl, "Distance"=w402:dbl)
                  n205 = In Range and Coerce(upper limit=405.0, x=w406, lower limit=395.0) -> (In Range?=w408:bool)  [unwired: 1 out]
                }
              }
              frame True {
                # "If it is within range, then the robot moves on to the shooting state"
              }
            }
            n206 = Negate(x=w374) -> (-x=w385:dbl)
            n207 = Less?(x=w373, y=w385) -> (x < y?=w386:bool)
            n208 = Select(t=w373, s=w386, f=w385) -> (s? t:f=w383:dbl)
          }
          frame "Shoot" {
            w439 = 0.0 ("LeftMotorsSpeed")
            # "If they weren't already, the motors of the drive are stopped."
            # "The robot then aligns itself vertically with the goal (also in pixels), charges up the shooting mechanism, and hopefully scores into the goal without problem"
            n209 = Unbundle By Name(w443) -> ("DriveRef"=w440:T2)
            n210 = call "Shoot.vi"("Trigger"=TRUE ("Collection Trigger"), "Vision Distance"=w441) -> ()  [unwired: 7 in, 3 out]
            n211 = call "Custom Tank.vi"("RobotDriveDevRef 2"=w440, "Left axis value"=w439, "Right axis value"=w439) -> ()  [unwired: 8 in, 5 out]
          }
          frame "Turn Back" {
            w450 = 0.0 ("New Sensor Position")
            # "The robot would then use the previously recorded value of rotation to align itself perpendicularly to the defense it came through"
            n212 = Unbundle By Name(w457) -> ("DriveRef"=w455:T2)
            n213 = Negate(x=w459) -> (-x=w460:dbl)
            n214 = call "Custom Tank.vi"("RobotDriveDevRef 2"=w455, "Left axis value"=-0.75 ("LeftMotorsSpeed"), "Right axis value"=0.75 ("RightMotorsSpeed")) -> ("Middle Left Motor"=w452:T3, "Middle Right Motor"=w451:T3)  [unwired: 8 in, 3 out]
            n215 = call <vilib>:"WPI_CANTalonSRX_SetSensorPosition.vi"("New Sensor Position"=w450, "CAN Talon SRX Ref"=w452) -> ("CAN Talon SRX Ref"=w449:T3)  [unwired: 8 in, 1 out]
            n216 = call <vilib>:"WPI_CANTalonSRX_SetSensorPosition.vi"("New Sensor Position"=w450, "CAN Talon SRX Ref"=w451) -> ("CAN Talon SRX Ref"=w448:T3)  [unwired: 8 in, 1 out]
            n217 = while {
              tunnel: w449 -> [w466]
              tunnel: w448 -> [w463]
              tunnel: w459 -> [w471]
              tunnel: w460 -> [w470]
              stop <- w472 stop-if-true
              n218 = call <vilib>:"WPI_CANTalonSRX_GetStatus.vi"("CAN Talon SRX Ref"=w466) -> ("Talon SRX Status"=w468:T15)  [unwired: 8 in, 2 out]
              n219 = call <vilib>:"WPI_CANTalonSRX_GetStatus.vi"("CAN Talon SRX Ref"=w463) -> ("Talon SRX Status"=w465:T15)  [unwired: 8 in, 2 out]
              n220 = Wait (ms)(milliseconds to wait=u32 20) -> ()  [unwired: 1 out]
              n221 = Unbundle By Name(w468) -> ("Encoder Position"=w467:dbl)
              n222 = Unbundle By Name(w465) -> ("Encoder Position"=w464:dbl)
              n223 = Less Or Equal?(x=w467, y=w470) -> (x <= y?=w474:bool)
              n224 = Greater Or Equal?(x=w464, y=w471) -> (x >= y?=w473:bool)
              n225 = And(x=w474, y=w473) -> (x .and. y?=w472:bool)
            }
          }
          frame "Move Back" {
            w479 = 0.0 ("New Sensor Position")
            w480 = -0.75 ("LeftMotorsSpeed")
            # "And then move back through the defense in order to get the next boulder as quickly as possible once Teleop starts."
            n226 = Unbundle By Name(w482) -> ("DriveRef"=w481:T2)
            n227 = call "Custom Tank.vi"("RobotDriveDevRef 2"=w481, "Left axis value"=w480, "Right axis value"=w480) -> ("Middle Left Motor"=w478:T3, "Middle Right Motor"=w477:T3)  [unwired: 8 in, 3 out]
            n228 = call <vilib>:"WPI_CANTalonSRX_SetSensorPosition.vi"("New Sensor Position"=w479, "CAN Talon SRX Ref"=w478) -> ("CAN Talon SRX Ref"=w476:T3)  [unwired: 8 in, 1 out]
            n229 = call <vilib>:"WPI_CANTalonSRX_SetSensorPosition.vi"("New Sensor Position"=w479, "CAN Talon SRX Ref"=w477) -> ("CAN Talon SRX Ref"=w475:T3)  [unwired: 8 in, 1 out]
            n230 = Negate(x=w484) -> (-x=w485:dbl)
            n231 = while {
              tunnel: w476 -> [w492]
              tunnel: w475 -> [w489]
              tunnel: w485 -> [w497]
              tunnel: w485 -> [w496]
              stop <- w498 stop-if-true
              n232 = call <vilib>:"WPI_CANTalonSRX_GetStatus.vi"("CAN Talon SRX Ref"=w492) -> ("Talon SRX Status"=w494:T15)  [unwired: 8 in, 2 out]
              n233 = call <vilib>:"WPI_CANTalonSRX_GetStatus.vi"("CAN Talon SRX Ref"=w489) -> ("Talon SRX Status"=w491:T15)  [unwired: 8 in, 2 out]
              n234 = Wait (ms)(milliseconds to wait=u32 20) -> ()  [unwired: 1 out]
              n235 = Unbundle By Name(w494) -> ("Encoder Position"=w493:dbl)
              n236 = Unbundle By Name(w491) -> ("Encoder Position"=w490:dbl)
              n237 = Less Or Equal?(x=w493, y=w497) -> (x <= y?=w500:bool)
              n238 = Less Or Equal?(x=w490, y=w496) -> (x <= y?=w499:bool)
              n239 = And(x=w500, y=w499) -> (x .and. y?=w498:bool)
            }
          }
          frame "End" {
            w501 = 0.0 ("New Sensor Position")
            w504 = 0.0 ("Left axis value")
            # "The autonomous is finished, the encoders are reset for the last time, and the loop stops, ending Autonomous."
            # "This is where autonomous ends"
            n240 = Unbundle By Name(w506) -> ("DriveRef"=w505:T2)
            n241 = call "Custom Tank.vi"("RobotDriveDevRef 2"=w505, "Left axis value"=w504, "Right axis value"=w504) -> ("Middle Left Motor"=w503:T3, "Middle Right Motor"=w502:T3)  [unwired: 8 in, 3 out]
            n242 = call <vilib>:"WPI_CANTalonSRX_SetSensorPosition.vi"("New Sensor Position"=w501, "CAN Talon SRX Ref"=w503) -> ()  [unwired: 8 in, 2 out]
            n243 = call <vilib>:"WPI_CANTalonSRX_SetSensorPosition.vi"("New Sensor Position"=w501, "CAN Talon SRX Ref"=w502) -> ()  [unwired: 8 in, 2 out]
          }
        }
      }
    }
    frame "Position 3" {
      w514 = 0.0  # Distance from the Goal (given by Vision)
      w515 = 0.0  # Rotation Distance
      w516 = 0.0  # Distance from Starting Point
      w517 = FALSE  # End loop?
      w518 = T16."Start"  # Beginning State
      # "Go through low bar, turn right until vision, shoot, return"
      n244 = while {
        shift-right: [w529] -> _
        shift-left: w518 -> [w530]
        shift-right: [w527] -> _
        shift-left: w517 -> [w528]
        shift-right: [w525] -> _
        shift-left: w516 -> [w526]
        shift-right: [w523] -> _
        shift-left: w515 -> [w524]
        shift-right: [w521] -> _
        shift-left: w514 -> [w522]
        tunnel: w513 -> [w520]
        tunnel: w512 -> [w519]
        stop <- w527 stop-if-true
        n245 = case shown="\"Start\", Default" w530 {
          tunnel: [w550 T16."Shoot" T16."Shoot" T16."Turn Back" T16."Move Back" T16."End" T16."End"] -> w529
          tunnel: [w549 w591 w632 w694 w709 w736 TRUE] -> w527
          tunnel: w528 -> [w549 w591 w632 w694 w709 w736 _]
          tunnel: [w543 w590 w631 w692 w708 w733 w759] -> w525
          tunnel: w526 -> [_ w590 w631 w692 w708 w733 w759]
          tunnel: w524 -> [w542 _ _ w691 w706 w735 w758]
          tunnel: [w542 w585 w628 w691 w706 w735 w758] -> w523
          tunnel: w522 -> [w541 _ _ w688 w705 w732 w757]
          tunnel: [w541 w583 w615 w688 w705 w732 w757] -> w521
          tunnel: w520 -> [w540 _ _ _ _ _ _]
          tunnel: w519 -> [w534 w582 w625 w690 w704 w731 w756]
          frame "Start", Default {
            w535 = 0.8 ("LeftMotorsSpeed")
            # "In order to prevent overshooting on the way back, the smaller distance recorded by\neither encoder would be kept."
            # "Stop the motors and bring the arms up 30 degrees so that they would see the goal better"
            # "Set the motors so the robot moves forward at moderate speed"
            # "Changes state depending on whether vision is needed (should be needed at least 99% of the time)"
            n246 = flat-sequence {
              tunnel: w534 -> [w551]
              tunnel: [w551] -> w533
              frame #0 {
                n247 = call "Zero Dart.vi"() -> ()  [unwired: 10 in, 2 out]
              }
            }
            n248 = Unbundle By Name(w533) -> ("DriveRef"=w536:T2)
            n249 = Select(t=T16."Turn (Vision)", s=w540, f=T16."Turn (No Vision)") -> (s? t:f=w550:T16)
            n250 = call "Custom Tank.vi"("RobotDriveDevRef 2"=w536, "Left axis value"=w535, "Right axis value"=w535) -> ("Middle Left Motor"=w532:T3, "Middle Right Motor"=w531:T3)  [unwired: 8 in, 3 out]
            n251 = while {
              tunnel: [w554] -> w538
              tunnel: [w555] -> w537
              tunnel: w533 -> [w558]
              tunnel: [w558] -> w539
              tunnel: w532 -> [w553]
              tunnel: w531 -> [w552]
              stop <- w563 stop-if-true
              # "The motors will continue running until both encoders meet the desired distance"
              n252 = call <vilib>:"WPI_CANTalonSRX_GetStatus.vi"("CAN Talon SRX Ref"=w553) -> ("Talon SRX Status"=w557:T15)  [unwired: 8 in, 2 out]
              n253 = call <vilib>:"WPI_CANTalonSRX_GetStatus.vi"("CAN Talon SRX Ref"=w552) -> ("Talon SRX Status"=w556:T15)  [unwired: 8 in, 2 out]
              n254 = Wait (ms)(milliseconds to wait=u32 20) -> ()  [unwired: 1 out]
              n255 = Unbundle By Name(w557) -> ("Encoder Position"=w554:dbl)
              n256 = Unbundle By Name(w556) -> ("Encoder Position"=w555:dbl)
              n257 = call "DistanceToEncoder.vi"("Gear Setting"=TRUE, "Distance (in)"=180.0 ("Distance")) -> ("Encoder Ticks"=w560:dbl)  [unwired: 9 in]
              n258 = Greater Or Equal?(x=w554, y=w560) -> (x >= y?=w565:bool)
              n259 = Greater Or Equal?(x=w555, y=w560) -> (x >= y?=w564:bool)
              n260 = And(x=w565, y=w564) -> (x .and. y?=w563:bool)
            }
            n261 = flat-sequence {
              tunnel: [w569] -> w545
              tunnel: [w568] -> w544
              tunnel: w539 -> [w570]
              tunnel: w538 -> [w569]
              tunnel: w537 -> [w568]
              frame #0 {
                w566 = 0.0 ("LeftMotorsSpeed")
                n262 = Unbundle By Name(w570) -> ("DriveRef"=w567:T2)
                n263 = call "Set Angle.vi"("Angle(degrees)"=60.0) -> ()  [unwired: 7 in, 4 out]
                n264 = Wait (ms)(milliseconds to wait=u32 2000) -> ()  [unwired: 1 out]
                n265 = call "Custom Tank.vi"("RobotDriveDevRef 2"=w567, "Left axis value"=w566, "Right axis value"=w566) -> ()  [unwired: 8 in, 5 out]
              }
            }
            n266 = Less?(x=w545, y=w544) -> (x < y?=w546:bool)
            n267 = Select(t=w545, s=w546, f=w544) -> (s? t:f=w543:dbl)
          }
          frame "Turn (No Vision)" {
            # "It is best not to use this code EVER!"
            # "Turn until certain encoder values are reached"
            n268 = Unbundle By Name(w582) -> ("DriveRef"=w581:T2)
            n269 = call "Custom Tank.vi"("RobotDriveDevRef 2"=w581, "Left axis value"=0.75 ("LeftMotorsSpeed"), "Right axis value"=-0.75 ("RightMotorsSpeed")) -> ("Middle Left Motor"=w574:T3, "Middle Right Motor"=w573:T3)  [unwired: 8 in, 3 out]
            n270 = call <vilib>:"WPI_CANTalonSRX_SetSensorPosition.vi"("New Sensor Position"=0.0, "CAN Talon SRX Ref"=w573) -> ("CAN Talon SRX Ref"=w576:T3)  [unwired: 8 in, 1 out]
            n271 = call <vilib>:"WPI_CANTalonSRX_SetSensorPosition.vi"("New Sensor Position"=0.0, "CAN Talon SRX Ref"=w574) -> ("CAN Talon SRX Ref"=w575:T3)  [unwired: 8 in, 1 out]
            n272 = while {
              tunnel: w575 -> [w594]
              tunnel: w576 -> [w593]
              tunnel: [w596] -> w587
              tunnel: [w595] -> w589
              stop <- w600 stop-if-true
              # "Replace 0s with actual values"
              n273 = call <vilib>:"WPI_CANTalonSRX_GetStatus.vi"("CAN Talon SRX Ref"=w594) -> ("Talon SRX Status"=w598:T15)  [unwired: 8 in, 2 out]
              n274 = call <vilib>:"WPI_CANTalonSRX_GetStatus.vi"("CAN Talon SRX Ref"=w593) -> ("Talon SRX Status"=w597:T15)  [unwired: 8 in, 2 out]
              n275 = Wait (ms)(milliseconds to wait=u32 20) -> ()  [unwired: 1 out]
              n276 = Unbundle By Name(w597) -> ("Encoder Position"=w595:dbl)
              n277 = Unbundle By Name(w598) -> ("Encoder Position"=w596:dbl)
              n278 = Less Or Equal?(x=w595, y=-0.0) -> (x <= y?=w602:bool)
              n279 = Greater Or Equal?(x=w596, y=0.0) -> (x >= y?=w603:bool)
              n280 = And(x=w603, y=w602) -> (x .and. y?=w600:bool)
            }
            n281 = Negate(x=w589) -> (-x=w586:dbl)
            n282 = Less?(x=w587, y=w586) -> (x < y?=w588:bool)
            n283 = Select(t=w587, s=w588, f=w586) -> (s? t:f=w585:dbl)
            n284 = global read "Robot Global Data.vi" "Vision Data"() -> (w584:T17)
            n285 = Unbundle By Name(w584) -> ("Distance"=w583:dbl)
          }
          frame "Turn (Vision)" {
            # "This turn goes on until the x-value of the center of the goal in pixels\nmatches the average x-value between the two (not displayed) cameras."
            # "Once again the smaller rotation distance of the two encoders\nare recorded, although one of them is reversed since it was going\nin reverse."
            # "Since the goal is towards the right, the robot will start turning in place"
            # "Both motors will stop and the robot checks if the goal is still centered within the range after half a second."
            n286 = Unbundle By Name(w625) -> ("DriveRef"=w613:T2)
            n287 = call "Custom Tank.vi"("RobotDriveDevRef 2"=w613, "Left axis value"=0.75 ("LeftMotorsSpeed"), "Right axis value"=-0.75 ("RightMotorsSpeed")) -> ("Middle Left Motor"=w606:T3, "Middle Right Motor"=w605:T3)  [unwired: 8 in, 3 out]
            n288 = call <vilib>:"WPI_CANTalonSRX_SetSensorPosition.vi"("New Sensor Position"=0.0, "CAN Talon SRX Ref"=w606) -> ("CAN Talon SRX Ref"=w608:T3)  [unwired: 8 in, 1 out]
            n289 = call <vilib>:"WPI_CANTalonSRX_SetSensorPosition.vi"("New Sensor Position"=0.0, "CAN Talon SRX Ref"=w605) -> ("CAN Talon SRX Ref"=w607:T3)  [unwired: 8 in, 1 out]
            n290 = while {
              tunnel: w607 -> [w659]
              tunnel: w608 -> [w660]
              tunnel: [w662] -> w626
              tunnel: [w661] -> w627
              stop <- w666 stop-if-true
              n291 = call <vilib>:"WPI_CANTalonSRX_GetStatus.vi"("CAN Talon SRX Ref"=w660) -> ("Talon SRX Status"=w664:T15)  [unwired: 8 in, 2 out]
              n292 = call <vilib>:"WPI_CANTalonSRX_GetStatus.vi"("CAN Talon SRX Ref"=w659) -> ("Talon SRX Status"=w663:T15)  [unwired: 8 in, 2 out]
              n293 = Wait (ms)(milliseconds to wait=u32 20) -> ()  [unwired: 1 out]
              n294 = Unbundle By Name(w664) -> ("Encoder Position"=w661:dbl)
              n295 = Unbundle By Name(w663) -> ("Encoder Position"=w662:dbl)
              n296 = global read "Robot Global Data.vi" "Vision Data"() -> (w670:T17)
              n297 = Unbundle By Name(w670) -> ("x"=w669:dbl)
              n298 = In Range and Coerce(upper limit=410.0, x=w669, lower limit=390.0) -> (In Range?=w666:bool)  [unwired: 1 out]
            }
            n299 = flat-sequence {
              tunnel: w627 -> [w674]
              tunnel: w626 -> [w673]
              tunnel: w625 -> [w675]
              tunnel: [w675] -> w619
              tunnel: [w674] -> w618
              tunnel: [w673] -> w617
              tunnel: [w683] -> w622
              tunnel: [w684] -> w623
              tunnel: [w685] -> w624
              tunnel: w619 -> [w685]
              tunnel: w618 -> [w684]
              tunnel: w617 -> [w683]
              tunnel: [w678] -> w616
              tunnel: [w677] -> w614
              frame #0 {
                w671 = 0.0 ("LeftMotorsSpeed")
                n300 = Unbundle By Name(w675) -> ("DriveRef"=w672:T2)
                n301 = Wait (ms)(milliseconds to wait=u32 500) -> ()  [unwired: 1 out]
                n302 = call "Custom Tank.vi"("RobotDriveDevRef 2"=w672, "Left axis value"=w671, "Right axis value"=w671) -> ()  [unwired: 8 in, 5 out]
              }
              frame #1 {
                n303 = global read "Robot Global Data.vi" "Vision Data"() -> (w682:T17)
                n304 = Unbundle By Name(w682) -> ("x"=w681:dbl, "Distance"=w677:dbl)
                n305 = In Range and Coerce(upper limit=410.0, x=w681, lower limit=390.0) -> (In Range?=w678:bool)  [unwired: 1 out]
              }
            }
            n306 = case shown="False" w616 {
              tunnel: [w641 w658] -> w620
              tunnel: w622 -> [_ w658]
              tunnel: w623 -> [_ w657]
              tunnel: [w642 w657] -> w621
              tunnel: w624 -> [w640 _]
              tunnel: [w639 w656] -> w615
              tunnel: w614 -> [_ w656]
              frame False {
                # "If it isn't within range then the robot will turn in place in the other direction at a slower pace until the desired pixel range is met"
                n307 = Unbundle By Name(w640) -> ("DriveRef"=w638:T2)
                n308 = call "Custom Tank.vi"("RobotDriveDevRef 2"=w638, "Left axis value"=-0.4 ("LeftMotorsSpeed"), "Right axis value"=0.4 ("RightMotorsSpeed")) -> ("Middle Left Motor"=w635:T3, "Middle Right Motor"=w634:T3)  [unwired: 8 in, 3 out]
                n309 = while {
                  tunnel: [w647] -> w642
                  tunnel: [w644] -> w641
                  tunnel: [w649] -> w639
                  tunnel: w635 -> [w646]
                  tunnel: w634 -> [w643]
                  stop <- w655 stop-if-true
                  n310 = call <vilib>:"WPI_CANTalonSRX_GetStatus.vi"("CAN Talon SRX Ref"=w646) -> ("Talon SRX Status"=w648:T15)  [unwired: 8 in, 2 out]
                  n311 = call <vilib>:"WPI_CANTalonSRX_GetStatus.vi"("CAN Talon SRX Ref"=w643) -> ("Talon SRX Status"=w645:T15)  [unwired: 8 in, 2 out]
                  n312 = Wait (ms)(milliseconds to wait=u32 20) -> ()  [unwired: 1 out]
                  n313 = Unbundle By Name(w648) -> ("Encoder Position"=w647:dbl)
                  n314 = Unbundle By Name(w645) -> ("Encoder Position"=w644:dbl)
                  n315 = global read "Robot Global Data.vi" "Vision Data"() -> (w654:T17)
                  n316 = Unbundle By Name(w654) -> ("x"=w653:dbl, "Distance"=w649:dbl)
                  n317 = In Range and Coerce(upper limit=405.0, x=w653, lower limit=395.0) -> (In Range?=w655:bool)  [unwired: 1 out]
                }
              }
              frame True {
                # "If it is within range, then the robot moves on to the shooting state"
              }
            }
            n318 = Negate(x=w620) -> (-x=w629:dbl)
            n319 = Less?(x=w621, y=w629) -> (x < y?=w630:bool)
            n320 = Select(t=w621, s=w630, f=w629) -> (s? t:f=w628:dbl)
          }
          frame "Shoot" {
            w686 = 0.0 ("LeftMotorsSpeed")
            # "If they weren't already, the motors of the drive are stopped."
            # "The robot then aligns itself vertically with the goal (also in pixels), charges up the shooting mechanism, and hopefully scores into the goal without problem"
            n321 = Unbundle By Name(w690) -> ("DriveRef"=w687:T2)
            n322 = call "Shoot.vi"("Trigger"=TRUE ("Collection Trigger"), "Vision Distance"=w688) -> ()  [unwired: 7 in, 3 out]
            n323 = call "Custom Tank.vi"("RobotDriveDevRef 2"=w687, "Left axis value"=w686, "Right axis value"=w686) -> ()  [unwired: 8 in, 5 out]
          }
          frame "Turn Back" {
            # "The robot would then use the previously recorded value of rotation to align itself perpendicularly to the defense it came through"
            n324 = Unbundle By Name(w704) -> ("DriveRef"=w703:T2)
            n325 = Negate(x=w706) -> (-x=w707:dbl)
            n326 = call "Custom Tank.vi"("RobotDriveDevRef 2"=w703, "Left axis value"=-0.75 ("LeftMotorsSpeed"), "Right axis value"=0.75 ("RightMotorsSpeed")) -> ("Middle Left Motor"=w696:T3, "Middle Right Motor"=w695:T3)  [unwired: 8 in, 3 out]
            n327 = call <vilib>:"WPI_CANTalonSRX_SetSensorPosition.vi"("New Sensor Position"=0.0, "CAN Talon SRX Ref"=w696) -> ("CAN Talon SRX Ref"=w697:T3)  [unwired: 8 in, 1 out]
            n328 = call <vilib>:"WPI_CANTalonSRX_SetSensorPosition.vi"("New Sensor Position"=0.0, "CAN Talon SRX Ref"=w695) -> ("CAN Talon SRX Ref"=w698:T3)  [unwired: 8 in, 1 out]
            n329 = while {
              tunnel: w697 -> [w712]
              tunnel: w698 -> [w711]
              tunnel: w706 -> [w719]
              tunnel: w707 -> [w718]
              stop <- w720 stop-if-true
              n330 = call <vilib>:"WPI_CANTalonSRX_GetStatus.vi"("CAN Talon SRX Ref"=w712) -> ("Talon SRX Status"=w716:T15)  [unwired: 8 in, 2 out]
              n331 = call <vilib>:"WPI_CANTalonSRX_GetStatus.vi"("CAN Talon SRX Ref"=w711) -> ("Talon SRX Status"=w714:T15)  [unwired: 8 in, 2 out]
              n332 = Wait (ms)(milliseconds to wait=u32 20) -> ()  [unwired: 1 out]
              n333 = Unbundle By Name(w716) -> ("Encoder Position"=w715:dbl)
              n334 = Unbundle By Name(w714) -> ("Encoder Position"=w713:dbl)
              n335 = Less Or Equal?(x=w715, y=w718) -> (x <= y?=w722:bool)
              n336 = Greater Or Equal?(x=w713, y=w719) -> (x >= y?=w721:bool)
              n337 = And(x=w722, y=w721) -> (x .and. y?=w720:bool)
            }
          }
          frame "Move Back" {
            w729 = -0.75 ("LeftMotorsSpeed")
            # "And then move back through the defense in order to get the next boulder as quickly as possible once Teleop starts."
            n338 = Unbundle By Name(w731) -> ("DriveRef"=w730:T2)
            n339 = call "Custom Tank.vi"("RobotDriveDevRef 2"=w730, "Left axis value"=w729, "Right axis value"=w729) -> ("Middle Left Motor"=w724:T3, "Middle Right Motor"=w723:T3)  [unwired: 8 in, 3 out]
            n340 = Negate(x=w733) -> (-x=w734:dbl)
            n341 = call <vilib>:"WPI_CANTalonSRX_SetSensorPosition.vi"("New Sensor Position"=0.0, "CAN Talon SRX Ref"=w724) -> ("CAN Talon SRX Ref"=w725:T3)  [unwired: 8 in, 1 out]
            n342 = call <vilib>:"WPI_CANTalonSRX_SetSensorPosition.vi"("New Sensor Position"=0.0, "CAN Talon SRX Ref"=w723) -> ("CAN Talon SRX Ref"=w726:T3)  [unwired: 8 in, 1 out]
            n343 = while {
              tunnel: w725 -> [w739]
              tunnel: w726 -> [w738]
              tunnel: w734 -> [w746]
              tunnel: w734 -> [w745]
              stop <- w747 stop-if-true
              n344 = call <vilib>:"WPI_CANTalonSRX_GetStatus.vi"("CAN Talon SRX Ref"=w739) -> ("Talon SRX Status"=w743:T15)  [unwired: 8 in, 2 out]
              n345 = call <vilib>:"WPI_CANTalonSRX_GetStatus.vi"("CAN Talon SRX Ref"=w738) -> ("Talon SRX Status"=w741:T15)  [unwired: 8 in, 2 out]
              n346 = Wait (ms)(milliseconds to wait=u32 20) -> ()  [unwired: 1 out]
              n347 = Unbundle By Name(w743) -> ("Encoder Position"=w742:dbl)
              n348 = Unbundle By Name(w741) -> ("Encoder Position"=w740:dbl)
              n349 = Less Or Equal?(x=w742, y=w746) -> (x <= y?=w749:bool)
              n350 = Less Or Equal?(x=w740, y=w745) -> (x <= y?=w748:bool)
              n351 = And(x=w749, y=w748) -> (x .and. y?=w747:bool)
            }
          }
          frame "End" {
            w754 = 0.0 ("Left axis value")
            # "The autonomous is finished, the encoders are reset for the last time, and the loop stops, ending Autonomous."
            n352 = Unbundle By Name(w756) -> ("DriveRef"=w755:T2)
            n353 = call "Custom Tank.vi"("RobotDriveDevRef 2"=w755, "Left axis value"=w754, "Right axis value"=w754) -> ("Middle Left Motor"=w751:T3, "Middle Right Motor"=w750:T3)  [unwired: 8 in, 3 out]
            n354 = call <vilib>:"WPI_CANTalonSRX_SetSensorPosition.vi"("New Sensor Position"=0.0, "CAN Talon SRX Ref"=w751) -> ()  [unwired: 8 in, 2 out]
            n355 = call <vilib>:"WPI_CANTalonSRX_SetSensorPosition.vi"("New Sensor Position"=0.0, "CAN Talon SRX Ref"=w750) -> ()  [unwired: 8 in, 2 out]
          }
        }
      }
    }
    frame "Position 4" {
      w763 = 0.0  # Distance from the Goal (given by Vision)
      w764 = 0.0  # Rotation Distance
      w765 = 0.0  # Distance from Starting Point
      w766 = FALSE  # End loop?
      w767 = T16."Start"  # Beginning State
      # "Go through low bar, turn right until vision, shoot, return"
      n356 = while {
        shift-right: [w777] -> _
        shift-left: w767 -> [w778]
        shift-right: [w775] -> _
        shift-left: w766 -> [w776]
        shift-right: [w773] -> _
        shift-left: w765 -> [w774]
        shift-right: [w771] -> _
        shift-left: w764 -> [w772]
        shift-right: [w769] -> _
        shift-left: w763 -> [w770]
        tunnel: w762 -> [w768]
        stop <- w775 stop-if-true
        n357 = case shown="\"Start\", Default" w778 {
          tunnel: [T16."Shoot" T16."Move Back" T16."End" T16."End"] -> w777
          tunnel: [w795 w828 w842 TRUE] -> w775
          tunnel: w776 -> [w795 w828 w842 _]
          tunnel: [w791 w826 w839 w865] -> w773
          tunnel: w774 -> [_ w826 w839 w865]
          tunnel: w772 -> [w790 w825 w841 w864]
          tunnel: [w790 w825 w841 w864] -> w771
          tunnel: w770 -> [_ w822 w838 w863]
          tunnel: [w785 w822 w838 w863] -> w769
          tunnel: w768 -> [w783 w824 w837 w862]
          frame "Start", Default {
            w781 = 0.8 ("LeftMotorsSpeed")
            # "In order to prevent overshooting on the way back, the smaller distance recorded by\neither encoder would be kept."
            # "Stop the motors and bring the arms up 30 degrees so that they would see the goal better"
            # "Set the motors so the robot moves forward at moderate speed"
            n358 = flat-sequence {
              tunnel: [w796] -> w784
              tunnel: w783 -> [w796]
              frame #0 {
                n359 = call "Zero Dart.vi"() -> ()  [unwired: 10 in, 2 out]
              }
            }
            n360 = Unbundle By Name(w784) -> ("DriveRef"=w782:T2)
            n361 = call "Custom Tank.vi"("RobotDriveDevRef 2"=w782, "Left axis value"=w781, "Right axis value"=w781) -> ("Middle Left Motor"=w780:T3, "Middle Right Motor"=w779:T3)  [unwired: 8 in, 3 out]
            n362 = while {
              tunnel: [w801] -> w788
              tunnel: [w799] -> w787
              tunnel: w784 -> [w803]
              tunnel: [w803] -> w786
              tunnel: w780 -> [w798]
              tunnel: w779 -> [w797]
              stop <- w808 stop-if-true
              # "The motors will continue running until both encoders meet the desired distance"
              n363 = call <vilib>:"WPI_CANTalonSRX_GetStatus.vi"("CAN Talon SRX Ref"=w797) -> ("Talon SRX Status"=w800:T15)  [unwired: 8 in, 2 out]
              n364 = Wait (ms)(milliseconds to wait=u32 20) -> ()  [unwired: 1 out]
              n365 = Unbundle By Name(w800) -> ("Encoder Position"=w799:dbl)
              n366 = call <vilib>:"WPI_CANTalonSRX_GetStatus.vi"("CAN Talon SRX Ref"=w798) -> ("Talon SRX Status"=w802:T15)  [unwired: 8 in, 2 out]
              n367 = Unbundle By Name(w802) -> ("Encoder Position"=w801:dbl)
              n368 = call "DistanceToEncoder.vi"("Gear Setting"=TRUE, "Distance (in)"=180.0 ("Distance")) -> ("Encoder Ticks"=w805:dbl)  [unwired: 9 in]
              n369 = Greater Or Equal?(x=w801, y=w805) -> (x >= y?=w810:bool)
              n370 = Greater Or Equal?(x=w799, y=w805) -> (x >= y?=w809:bool)
              n371 = And(x=w810, y=w809) -> (x .and. y?=w808:bool)
            }
            n372 = flat-sequence {
              tunnel: [w817] -> w793
              tunnel: [w816] -> w792
              tunnel: w788 -> [w817]
              tunnel: w787 -> [w816]
              tunnel: w786 -> [w815]
              tunnel: [w813] -> w785
              frame #0 {
                w811 = 0.0 ("LeftMotorsSpeed")
                n373 = Unbundle By Name(w815) -> ("DriveRef"=w812:T2)
                n374 = call "Set Angle.vi"("Angle(degrees)"=60.0) -> ()  [unwired: 7 in, 4 out]
                n375 = Wait (ms)(milliseconds to wait=u32 2000) -> ()  [unwired: 1 out]
                n376 = call "Custom Tank.vi"("RobotDriveDevRef 2"=w812, "Left axis value"=w811, "Right axis value"=w811) -> ()  [unwired: 8 in, 5 out]
                n377 = global read "Robot Global Data.vi" "Vision Data"() -> (w814:T17)
                n378 = Unbundle By Name(w814) -> ("Distance"=w813:dbl)
              }
            }
            n379 = Less?(x=w793, y=w792) -> (x < y?=w794:bool)
            n380 = Select(t=w793, s=w794, f=w792) -> (s? t:f=w791:dbl)
          }
          frame "Shoot" {
            w820 = 0.0 ("LeftMotorsSpeed")
            # "If they weren't already, the motors of the drive are stopped."
            # "The robot then aligns itself vertically with the goal (also in pixels), charges up the shooting mechanism, and hopefully scores into the goal without problem"
            # "Shoot the boulder"
            n381 = Unbundle By Name(w824) -> ("DriveRef"=w821:T2)
            n382 = call "Shoot.vi"("Trigger"=TRUE ("Collection Trigger"), "Vision Distance"=w822) -> ()  [unwired: 7 in, 3 out]
            n383 = call "Custom Tank.vi"("RobotDriveDevRef 2"=w821, "Left axis value"=w820, "Right axis value"=w820) -> ()  [unwired: 8 in, 5 out]
          }
          frame "Move Back" {
            w835 = -0.75 ("LeftMotorsSpeed")
            # "The robot would then use the previously recorded distance to  move back through the defense in order to get the next boulder as quickly as possible once Teleop starts."
            n384 = Unbundle By Name(w837) -> ("DriveRef"=w836:T2)
            n385 = call "Custom Tank.vi"("RobotDriveDevRef 2"=w836, "Left axis value"=w835, "Right axis value"=w835) -> ("Middle Left Motor"=w832:T3, "Middle Right Motor"=w831:T3)  [unwired: 8 in, 3 out]
            n386 = Negate(x=w839) -> (-x=w840:dbl)
            n387 = call <vilib>:"WPI_CANTalonSRX_SetSensorPosition.vi"("New Sensor Position"=0.0, "CAN Talon SRX Ref"=w832) -> ("CAN Talon SRX Ref"=w830:T3)  [unwired: 8 in, 1 out]
            n388 = call <vilib>:"WPI_CANTalonSRX_SetSensorPosition.vi"("New Sensor Position"=0.0, "CAN Talon SRX Ref"=w831) -> ("CAN Talon SRX Ref"=w829:T3)  [unwired: 8 in, 1 out]
            n389 = while {
              tunnel: w830 -> [w847]
              tunnel: w829 -> [w844]
              tunnel: w840 -> [w852]
              tunnel: w840 -> [w851]
              stop <- w853 stop-if-true
              n390 = call <vilib>:"WPI_CANTalonSRX_GetStatus.vi"("CAN Talon SRX Ref"=w847) -> ("Talon SRX Status"=w849:T15)  [unwired: 8 in, 2 out]
              n391 = call <vilib>:"WPI_CANTalonSRX_GetStatus.vi"("CAN Talon SRX Ref"=w844) -> ("Talon SRX Status"=w846:T15)  [unwired: 8 in, 2 out]
              n392 = Wait (ms)(milliseconds to wait=u32 20) -> ()  [unwired: 1 out]
              n393 = Unbundle By Name(w849) -> ("Encoder Position"=w848:dbl)
              n394 = Unbundle By Name(w846) -> ("Encoder Position"=w845:dbl)
              n395 = Less Or Equal?(x=w848, y=w852) -> (x <= y?=w855:bool)
              n396 = Less Or Equal?(x=w845, y=w851) -> (x <= y?=w854:bool)
              n397 = And(x=w855, y=w854) -> (x .and. y?=w853:bool)
            }
          }
          frame "End" {
            w861 = 0.0 ("Left axis value")
            # "The autonomous is finished, the encoders are reset for the last time, and the loop stops, ending Autonomous."
            n398 = Unbundle By Name(w862) -> ("DriveRef"=w858:T2)
            n399 = call "Custom Tank.vi"("RobotDriveDevRef 2"=w858, "Left axis value"=w861, "Right axis value"=w861) -> ("Middle Left Motor"=w857:T3, "Middle Right Motor"=w856:T3)  [unwired: 8 in, 3 out]
            n400 = call <vilib>:"WPI_CANTalonSRX_SetSensorPosition.vi"("New Sensor Position"=0.0, "CAN Talon SRX Ref"=w857) -> ()  [unwired: 8 in, 2 out]
            n401 = call <vilib>:"WPI_CANTalonSRX_SetSensorPosition.vi"("New Sensor Position"=0.0, "CAN Talon SRX Ref"=w856) -> ()  [unwired: 8 in, 2 out]
          }
        }
      }
    }
    frame "Position 5" {
      w871 = 0.0  # Distance from the Goal (given by Vision)
      w872 = 0.0  # Rotation Distance
      w870 = 0.0  # Distance from Starting Point
      w873 = FALSE  # End loop?
      w874 = T16."Start"  # Beginning State
      # "Go through low bar, turn left until vision, shoot, return"
      n402 = while {
        shift-right: [w885] -> _
        shift-left: w874 -> [w886]
        shift-right: [w883] -> _
        shift-left: w873 -> [w884]
        shift-right: [w881] -> _
        shift-left: w870 -> [w882]
        shift-right: [w879] -> _
        shift-left: w872 -> [w880]
        shift-right: [w877] -> _
        shift-left: w871 -> [w878]
        tunnel: w869 -> [w876]
        tunnel: w868 -> [w875]
        stop <- w883 stop-if-true
        n403 = case shown="\"Start\", Default" w886 {
          tunnel: [w906 T16."Shoot" T16."Shoot" T16."Turn Back" T16."Move Back" T16."End" T16."End"] -> w885
          tunnel: [w905 w947 w989 w1052 w1067 w1094 TRUE] -> w883
          tunnel: w884 -> [w905 w947 w989 w1052 w1067 w1094 _]
          tunnel: [w899 w946 w988 w1050 w1066 w1091 w1117] -> w881
          tunnel: w882 -> [_ w946 w988 w1050 w1066 w1091 w1117]
          tunnel: w880 -> [w898 _ _ w1049 w1064 w1093 w1116]
          tunnel: [w898 w941 w985 w1049 w1064 w1093 w1116] -> w879
          tunnel: w878 -> [w897 _ _ w1046 w1063 w1090 w1115]
          tunnel: [w897 w939 w971 w1046 w1063 w1090 w1115] -> w877
          tunnel: w876 -> [w896 _ _ _ _ _ _]
          tunnel: w875 -> [w891 w938 w980 w1048 w1062 w1089 w1114]
          frame "Start", Default {
            w889 = 0.8 ("LeftMotorsSpeed")
            # "In order to prevent overshooting on the way back, the smaller distance recorded by\neither encoder would be kept."
            # "Stop the motors and bring the arms up 30 degrees so that they would see the goal better"
            # "Set the motors so the robot moves forward at moderate speed"
            # "Changes state depending on whether vision is needed (should be needed at least 99% of the time)"
            n404 = flat-sequence {
              tunnel: w891 -> [w907]
              tunnel: [w907] -> w892
              frame #0 {
                n405 = call "Zero Dart.vi"() -> ()  [unwired: 10 in, 2 out]
              }
            }
            n406 = Unbundle By Name(w892) -> ("DriveRef"=w890:T2)
            n407 = Select(t=T16."Turn (Vision)", s=w896, f=T16."Turn (No Vision)") -> (s? t:f=w906:T16)
            n408 = call "Custom Tank.vi"("RobotDriveDevRef 2"=w890, "Left axis value"=w889, "Right axis value"=w889) -> ("Middle Left Motor"=w888:T3, "Middle Right Motor"=w887:T3)  [unwired: 8 in, 3 out]
            n409 = while {
              tunnel: [w911] -> w894
              tunnel: [w909] -> w895
              tunnel: w892 -> [w915]
              tunnel: [w915] -> w893
              tunnel: w888 -> [w912]
              tunnel: w887 -> [w908]
              stop <- w919 stop-if-true
              # "The motors will continue running until both encoders meet the desired distance"
              n410 = call <vilib>:"WPI_CANTalonSRX_GetStatus.vi"("CAN Talon SRX Ref"=w912) -> ("Talon SRX Status"=w913:T15)  [unwired: 8 in, 2 out]
              n411 = call <vilib>:"WPI_CANTalonSRX_GetStatus.vi"("CAN Talon SRX Ref"=w908) -> ("Talon SRX Status"=w910:T15)  [unwired: 8 in, 2 out]
              n412 = Wait (ms)(milliseconds to wait=u32 20) -> ()  [unwired: 1 out]
              n413 = Unbundle By Name(w913) -> ("Encoder Position"=w911:dbl)
              n414 = Unbundle By Name(w910) -> ("Encoder Position"=w909:dbl)
              n415 = call "DistanceToEncoder.vi"("Gear Setting"=TRUE, "Distance (in)"=180.0 ("Distance")) -> ("Encoder Ticks"=w916:dbl)  [unwired: 9 in]
              n416 = Greater Or Equal?(x=w911, y=w916) -> (x >= y?=w921:bool)
              n417 = Greater Or Equal?(x=w909, y=w916) -> (x >= y?=w920:bool)
              n418 = And(x=w921, y=w920) -> (x .and. y?=w919:bool)
            }
            n419 = flat-sequence {
              tunnel: [w925] -> w901
              tunnel: [w926] -> w900
              tunnel: w895 -> [w926]
              tunnel: w894 -> [w925]
              tunnel: w893 -> [w924]
              frame #0 {
                w923 = 0.0 ("LeftMotorsSpeed")
                # "Bring the arms up to a certain angle in order to see the goal later"
                n420 = Unbundle By Name(w924) -> ("DriveRef"=w922:T2)
                n421 = call "Set Angle.vi"("Angle(degrees)"=60.0) -> ()  [unwired: 7 in, 4 out]
                n422 = Wait (ms)(milliseconds to wait=u32 2000) -> ()  [unwired: 1 out]
                n423 = call "Custom Tank.vi"("RobotDriveDevRef 2"=w922, "Left axis value"=w923, "Right axis value"=w923) -> ()  [unwired: 8 in, 5 out]
              }
            }
            n424 = Less?(x=w901, y=w900) -> (x < y?=w902:bool)
            n425 = Select(t=w901, s=w902, f=w900) -> (s? t:f=w899:dbl)
          }
          frame "Turn (No Vision)" {
            # "It is best not to use this code EVER!"
            # "Turn until certain encoder values are reached"
            n426 = Unbundle By Name(w938) -> ("DriveRef"=w937:T2)
            n427 = call "Custom Tank.vi"("RobotDriveDevRef 2"=w937, "Left axis value"=-0.75 ("LeftMotorsSpeed"), "Right axis value"=0.75 ("RightMotorsSpeed")) -> ("Middle Left Motor"=w933:T3, "Middle Right Motor"=w931:T3)  [unwired: 8 in, 3 out]
            n428 = call <vilib>:"WPI_CANTalonSRX_SetSensorPosition.vi"("New Sensor Position"=0.0, "CAN Talon SRX Ref"=w933) -> ("CAN Talon SRX Ref"=w930:T3)  [unwired: 8 in, 1 out]
            n429 = call <vilib>:"WPI_CANTalonSRX_SetSensorPosition.vi"("New Sensor Position"=0.0, "CAN Talon SRX Ref"=w931) -> ("CAN Talon SRX Ref"=w929:T3)  [unwired: 8 in, 1 out]
            n430 = while {
              tunnel: w929 -> [w950]
              tunnel: w930 -> [w949]
              tunnel: [w951] -> w943
              tunnel: [w953] -> w945
              stop <- w956 stop-if-true
              # "Replace 0s with actual values"
              n431 = call <vilib>:"WPI_CANTalonSRX_GetStatus.vi"("CAN Talon SRX Ref"=w949) -> ("Talon SRX Status"=w954:T15)  [unwired: 8 in, 2 out]
              n432 = call <vilib>:"WPI_CANTalonSRX_GetStatus.vi"("CAN Talon SRX Ref"=w950) -> ("Talon SRX Status"=w952:T15)  [unwired: 8 in, 2 out]
              n433 = Wait (ms)(milliseconds to wait=u32 20) -> ()  [unwired: 1 out]
              n434 = Unbundle By Name(w952) -> ("Encoder Position"=w951:dbl)
              n435 = Unbundle By Name(w954) -> ("Encoder Position"=w953:dbl)
              n436 = Greater Or Equal?(x=w951, y=0.0) -> (x >= y?=w959:bool)
              n437 = Less Or Equal?(x=w953, y=-0.0) -> (x <= y?=w958:bool)
              n438 = And(x=w959, y=w958) -> (x .and. y?=w956:bool)
            }
            n439 = Negate(x=w945) -> (-x=w942:dbl)
            n440 = Less?(x=w943, y=w942) -> (x < y?=w944:bool)
            n441 = Select(t=w943, s=w944, f=w942) -> (s? t:f=w941:dbl)
            n442 = global read "Robot Global Data.vi" "Vision Data"() -> (w940:T17)
            n443 = Unbundle By Name(w940) -> ("Distance"=w939:dbl)
          }
          frame "Turn (Vision)" {
            # "Once again the smaller rotation distance of the two encoders\nare recorded, although one of them is reversed since it was going\nin reverse."
            # "Both motors will stop and the robot checks if the goal is still centered within the range after half a second."
            # "This turn goes on until the x-value of the center of the goal in pixels\nmatches the average x-value between the two (not displayed) cameras."
            # "Since the goal is towards the left, the robot will start turning in place"
            n444 = Unbundle By Name(w980) -> ("DriveRef"=w969:T2)
            n445 = call "Custom Tank.vi"("RobotDriveDevRef 2"=w969, "Left axis value"=-0.75 ("LeftMotorsSpeed"), "Right axis value"=0.75 ("RightMotorsSpeed")) -> ("Middle Left Motor"=w964:T3, "Middle Right Motor"=w963:T3)  [unwired: 8 in, 3 out]
            n446 = call <vilib>:"WPI_CANTalonSRX_SetSensorPosition.vi"("New Sensor Position"=0.0, "CAN Talon SRX Ref"=w964) -> ("CAN Talon SRX Ref"=w962:T3)  [unwired: 8 in, 1 out]
            n447 = call <vilib>:"WPI_CANTalonSRX_SetSensorPosition.vi"("New Sensor Position"=0.0, "CAN Talon SRX Ref"=w963) -> ("CAN Talon SRX Ref"=w961:T3)  [unwired: 8 in, 1 out]
            n448 = while {
              tunnel: w962 -> [w1019]
              tunnel: w961 -> [w1018]
              tunnel: [w1017] -> w981
              tunnel: [w1016] -> w982
              tunnel: w980 -> [w1022]
              tunnel: [w1022] -> w979
              stop <- w1028 stop-if-true
              n449 = call <vilib>:"WPI_CANTalonSRX_GetStatus.vi"("CAN Talon SRX Ref"=w1019) -> ("Talon SRX Status"=w1021:T15)  [unwired: 8 in, 2 out]
              n450 = call <vilib>:"WPI_CANTalonSRX_GetStatus.vi"("CAN Talon SRX Ref"=w1018) -> ("Talon SRX Status"=w1020:T15)  [unwired: 8 in, 2 out]
              n451 = Wait (ms)(milliseconds to wait=u32 20) -> ()  [unwired: 1 out]
              n452 = Unbundle By Name(w1021) -> ("Encoder Position"=w1017:dbl)
              n453 = Unbundle By Name(w1020) -> ("Encoder Position"=w1016:dbl)
              n454 = global read "Robot Global Data.vi" "Vision Data"() -> (w1027:T17)
              n455 = Unbundle By Name(w1027) -> ("x"=w1026:dbl)
              n456 = In Range and Coerce(upper limit=410.0, x=w1026, lower limit=390.0) -> (In Range?=w1028:bool)  [unwired: 1 out]
            }
            n457 = flat-sequence {
              tunnel: [w1032] -> w984
              tunnel: [w1033] -> w983
              tunnel: w982 -> [w1033]
              tunnel: w981 -> [w1032]
              tunnel: w979 -> [w1031]
              tunnel: [w1031] -> w978
              tunnel: w984 -> [w1038]
              tunnel: w983 -> [w1037]
              tunnel: w978 -> [w1039]
              tunnel: [w1039] -> w977
              tunnel: [w1038] -> w976
              tunnel: [w1037] -> w975
              tunnel: [w1036] -> w972
              tunnel: [w1035] -> w970
              frame #0 {
                w1029 = 0.0 ("LeftMotorsSpeed")
                n458 = Unbundle By Name(w1031) -> ("DriveRef"=w1030:T2)
                n459 = Wait (ms)(milliseconds to wait=u32 500) -> ()  [unwired: 1 out]
                n460 = call "Custom Tank.vi"("RobotDriveDevRef 2"=w1030, "Left axis value"=w1029, "Right axis value"=w1029) -> ()  [unwired: 8 in, 5 out]
              }
              frame #1 {
                n461 = global read "Robot Global Data.vi" "Vision Data"() -> (w1043:T17)
                n462 = Unbundle By Name(w1043) -> ("x"=w1042:dbl, "Distance"=w1035:dbl)
                n463 = In Range and Coerce(upper limit=410.0, x=w1042, lower limit=390.0) -> (In Range?=w1036:bool)  [unwired: 1 out]
              }
            }
            n464 = case shown="False" w972 {
              tunnel: [w998 w1015] -> w973
              tunnel: w975 -> [_ w1015]
              tunnel: w976 -> [_ w1014]
              tunnel: [w999 w1014] -> w974
              tunnel: w977 -> [w997 _]
              tunnel: [w996 w1013] -> w971
              tunnel: w970 -> [_ w1013]
              frame False {
                # "If it isn't within range then the robot will turn in place in the other direction at a slower pace until the desired pixel range is met"
                n465 = Unbundle By Name(w997) -> ("DriveRef"=w995:T2)
                n466 = call "Custom Tank.vi"("RobotDriveDevRef 2"=w995, "Left axis value"=0.4 ("LeftMotorsSpeed"), "Right axis value"=-0.4 ("RightMotorsSpeed")) -> ("Middle Left Motor"=w992:T3, "Middle Right Motor"=w991:T3)  [unwired: 8 in, 3 out]
                n467 = while {
                  tunnel: [w1004] -> w999
                  tunnel: [w1002] -> w998
                  tunnel: [w1006] -> w996
                  tunnel: w992 -> [w1001]
                  tunnel: w991 -> [w1000]
                  stop <- w1012 stop-if-true
                  n468 = call <vilib>:"WPI_CANTalonSRX_GetStatus.vi"("CAN Talon SRX Ref"=w1001) -> ("Talon SRX Status"=w1005:T15)  [unwired: 8 in, 2 out]
                  n469 = call <vilib>:"WPI_CANTalonSRX_GetStatus.vi"("CAN Talon SRX Ref"=w1000) -> ("Talon SRX Status"=w1003:T15)  [unwired: 8 in, 2 out]
                  n470 = Wait (ms)(milliseconds to wait=u32 20) -> ()  [unwired: 1 out]
                  n471 = Unbundle By Name(w1005) -> ("Encoder Position"=w1004:dbl)
                  n472 = Unbundle By Name(w1003) -> ("Encoder Position"=w1002:dbl)
                  n473 = global read "Robot Global Data.vi" "Vision Data"() -> (w1011:T17)
                  n474 = Unbundle By Name(w1011) -> ("x"=w1010:dbl, "Distance"=w1006:dbl)
                  n475 = In Range and Coerce(upper limit=405.0, x=w1010, lower limit=395.0) -> (In Range?=w1012:bool)  [unwired: 1 out]
                }
              }
              frame True {
                # "If it is within range, then the robot moves on to the shooting state"
              }
            }
            n476 = Negate(x=w974) -> (-x=w986:dbl)
            n477 = Less?(x=w973, y=w986) -> (x < y?=w987:bool)
            n478 = Select(t=w973, s=w987, f=w986) -> (s? t:f=w985:dbl)
          }
          frame "Shoot" {
            w1044 = 0.0 ("LeftMotorsSpeed")
            # "If they weren't already, the motors of the drive are stopped."
            # "The robot then aligns itself vertically with the goal (also in pixels), charges up the shooting mechanism, and hopefully scores into the goal without problem"
            n479 = Unbundle By Name(w1048) -> ("DriveRef"=w1045:T2)
            n480 = call "Shoot.vi"("Trigger"=TRUE ("Collection Trigger"), "Vision Distance"=w1046) -> ()  [unwired: 7 in, 3 out]
            n481 = call "Custom Tank.vi"("RobotDriveDevRef 2"=w1045, "Left axis value"=w1044, "Right axis value"=w1044) -> ()  [unwired: 8 in, 5 out]
          }
          frame "Turn Back" {
            # "The robot would then use the previously recorded value of rotation to align itself perpendicularly to the defense it came through"
            n482 = Unbundle By Name(w1062) -> ("DriveRef"=w1061:T2)
            n483 = Negate(x=w1064) -> (-x=w1065:dbl)
            n484 = call "Custom Tank.vi"("RobotDriveDevRef 2"=w1061, "Left axis value"=0.75 ("LeftMotorsSpeed"), "Right axis value"=-0.75 ("RightMotorsSpeed")) -> ("Middle Left Motor"=w1056:T3, "Middle Right Motor"=w1055:T3)  [unwired: 8 in, 3 out]
            n485 = call <vilib>:"WPI_CANTalonSRX_SetSensorPosition.vi"("New Sensor Position"=0.0, "CAN Talon SRX Ref"=w1056) -> ("CAN Talon SRX Ref"=w1053:T3)  [unwired: 8 in, 1 out]
            n486 = call <vilib>:"WPI_CANTalonSRX_SetSensorPosition.vi"("New Sensor Position"=0.0, "CAN Talon SRX Ref"=w1055) -> ("CAN Talon SRX Ref"=w1054:T3)  [unwired: 8 in, 1 out]
            n487 = while {
              tunnel: w1054 -> [w1070]
              tunnel: w1053 -> [w1069]
              tunnel: w1064 -> [w1077]
              tunnel: w1065 -> [w1076]
              stop <- w1078 stop-if-true
              n488 = call <vilib>:"WPI_CANTalonSRX_GetStatus.vi"("CAN Talon SRX Ref"=w1069) -> ("Talon SRX Status"=w1074:T15)  [unwired: 8 in, 2 out]
              n489 = call <vilib>:"WPI_CANTalonSRX_GetStatus.vi"("CAN Talon SRX Ref"=w1070) -> ("Talon SRX Status"=w1072:T15)  [unwired: 8 in, 2 out]
              n490 = Wait (ms)(milliseconds to wait=u32 20) -> ()  [unwired: 1 out]
              n491 = Unbundle By Name(w1074) -> ("Encoder Position"=w1073:dbl)
              n492 = Unbundle By Name(w1072) -> ("Encoder Position"=w1071:dbl)
              n493 = Less Or Equal?(x=w1071, y=w1076) -> (x <= y?=w1080:bool)
              n494 = Greater Or Equal?(x=w1073, y=w1077) -> (x >= y?=w1079:bool)
              n495 = And(x=w1080, y=w1079) -> (x .and. y?=w1078:bool)
            }
          }
          frame "Move Back" {
            w1087 = -0.75 ("LeftMotorsSpeed")
            # "The robot would then use the previously recorded distance to  move back through the defense in order to get the next boulder as quickly as possible once Teleop starts."
            n496 = Unbundle By Name(w1089) -> ("DriveRef"=w1088:T2)
            n497 = call "Custom Tank.vi"("RobotDriveDevRef 2"=w1088, "Left axis value"=w1087, "Right axis value"=w1087) -> ("Middle Left Motor"=w1085:T3, "Middle Right Motor"=w1083:T3)  [unwired: 8 in, 3 out]
            n498 = Negate(x=w1091) -> (-x=w1092:dbl)
            n499 = call <vilib>:"WPI_CANTalonSRX_SetSensorPosition.vi"("New Sensor Position"=0.0, "CAN Talon SRX Ref"=w1085) -> ("CAN Talon SRX Ref"=w1082:T3)  [unwired: 8 in, 1 out]
            n500 = call <vilib>:"WPI_CANTalonSRX_SetSensorPosition.vi"("New Sensor Position"=0.0, "CAN Talon SRX Ref"=w1083) -> ("CAN Talon SRX Ref"=w1081:T3)  [unwired: 8 in, 1 out]
            n501 = while {
              tunnel: w1082 -> [w1097]
              tunnel: w1081 -> [w1096]
              tunnel: w1092 -> [w1104]
              tunnel: w1092 -> [w1103]
              stop <- w1105 stop-if-true
              # "Move back to start"
              n502 = call <vilib>:"WPI_CANTalonSRX_GetStatus.vi"("CAN Talon SRX Ref"=w1097) -> ("Talon SRX Status"=w1101:T15)  [unwired: 8 in, 2 out]
              n503 = call <vilib>:"WPI_CANTalonSRX_GetStatus.vi"("CAN Talon SRX Ref"=w1096) -> ("Talon SRX Status"=w1099:T15)  [unwired: 8 in, 2 out]
              n504 = Wait (ms)(milliseconds to wait=u32 20) -> ()  [unwired: 1 out]
              n505 = Unbundle By Name(w1101) -> ("Encoder Position"=w1100:dbl)
              n506 = Unbundle By Name(w1099) -> ("Encoder Position"=w1098:dbl)
              n507 = Less Or Equal?(x=w1100, y=w1104) -> (x <= y?=w1107:bool)
              n508 = Less Or Equal?(x=w1098, y=w1103) -> (x <= y?=w1106:bool)
              n509 = And(x=w1107, y=w1106) -> (x .and. y?=w1105:bool)
            }
          }
          frame "End" {
            w1112 = 0.0 ("Left axis value")
            # "The autonomous is finished, the encoders are reset for the last time, and the loop stops, ending Autonomous."
            n510 = Unbundle By Name(w1114) -> ("DriveRef"=w1113:T2)
            n511 = call "Custom Tank.vi"("RobotDriveDevRef 2"=w1113, "Left axis value"=w1112, "Right axis value"=w1112) -> ("Middle Left Motor"=w1109:T3, "Middle Right Motor"=w1108:T3)  [unwired: 8 in, 3 out]
            n512 = call <vilib>:"WPI_CANTalonSRX_SetSensorPosition.vi"("New Sensor Position"=0.0, "CAN Talon SRX Ref"=w1109) -> ()  [unwired: 8 in, 2 out]
            n513 = call <vilib>:"WPI_CANTalonSRX_SetSensorPosition.vi"("New Sensor Position"=0.0, "CAN Talon SRX Ref"=w1108) -> ()  [unwired: 8 in, 2 out]
          }
        }
      }
    }
    frame "Move Forward at Dist. Test" {
      n514 = flat-sequence {
        tunnel: w1120 -> [w1126]
        tunnel: [w1127] -> w1121
        tunnel: w1121 -> [w1149]
        frame #0 {
          w1124 = 0.8 ("LeftMotorsSpeed")
          # "Set the motors so the robot moves forward at moderate speed"
          n515 = Unbundle By Name(w1126) -> ("DriveRef"=w1125:T2)
          n516 = call "Custom Tank.vi"("RobotDriveDevRef 2"=w1125, "Left axis value"=w1124, "Right axis value"=w1124) -> ("Middle Left Motor"=w1123:T3, "Middle Right Motor"=w1122:T3)  [unwired: 8 in, 3 out]
          n517 = while {
            tunnel: [w1132] -> _
            tunnel: [w1130] -> _
            tunnel: [w1135] -> w1127
            tunnel: w1126 -> [w1135]
            tunnel: w1123 -> [w1129]
            tunnel: w1122 -> [w1128]
            stop <- w1139 stop-if-true
            # "The motors will continue running until both encoders meet the desired distance"
            n518 = call <vilib>:"WPI_CANTalonSRX_GetStatus.vi"("CAN Talon SRX Ref"=w1129) -> ("Talon SRX Status"=w1133:T15)  [unwired: 8 in, 2 out]
            n519 = call <vilib>:"WPI_CANTalonSRX_GetStatus.vi"("CAN Talon SRX Ref"=w1128) -> ("Talon SRX Status"=w1131:T15)  [unwired: 8 in, 2 out]
            n520 = Wait (ms)(milliseconds to wait=u32 20) -> ()  [unwired: 1 out]
            n521 = Unbundle By Name(w1133) -> ("Encoder Position"=w1132:dbl)
            n522 = Unbundle By Name(w1131) -> ("Encoder Position"=w1130:dbl)
            n523 = call "DistanceToEncoder.vi"("Gear Setting"="Gear Setting", "Distance (in)"="Distance (in)") -> ("Encoder Ticks"=w1137:dbl)  [unwired: 9 in]
            n524 = Greater Or Equal?(x=w1132, y=w1137) -> (x >= y?=w1141:bool)
            n525 = Greater Or Equal?(x=w1130, y=w1137) -> (x >= y?=w1140:bool)
            n526 = And(x=w1141, y=w1140) -> (x .and. y?=w1139:bool)
          }
        }
        frame #1 {
          w1146 = 0.0 ("LeftMotorsSpeed")
          n527 = Unbundle By Name(w1149) -> ("DriveRef"=w1147:T2)
          n528 = call "Custom Tank.vi"("RobotDriveDevRef 2"=w1147, "Left axis value"=w1146, "Right axis value"=w1146) -> ("Middle Left Motor"=w1143:T3, "Middle Right Motor"=w1142:T3)  [unwired: 8 in, 3 out]
          n529 = call <vilib>:"WPI_CANTalonSRX_SetSensorPosition.vi"("New Sensor Position"=0.0, "CAN Talon SRX Ref"=w1143) -> ()  [unwired: 8 in, 2 out]
          n530 = call <vilib>:"WPI_CANTalonSRX_SetSensorPosition.vi"("New Sensor Position"=0.0, "CAN Talon SRX Ref"=w1142) -> ()  [unwired: 8 in, 2 out]
          "End?" <- TRUE ("Success?")
        }
      }
    }
    frame "Turn Until Vision Test" {
      w1150 = T16."Turn (Vision)"  # Beginning State
      n531 = case shown="\"Turn (Vision)\"" w1150 {
        tunnel: w1151 -> [_ _ w1170 _ _ _ _]
        frame "Start", Default {
        }
        frame "Turn (No Vision)" {
          (unwired) T16."Shoot"
          n532 = global read "Robot Global Data.vi" "Vision Data"() -> (w1152:T17)
          n533 = Unbundle By Name(w1152) -> ()  [unwired: 1 out]
        }
        frame "Turn (Vision)" {
          # "Both motors will stop and the robot checks if the goal is still centered within the range after half a second."
          # "This turn goes on until the x-value of the center of the goal in pixels\nmatches the average x-value between the two (not displayed) cameras."
          # "Since the goal is towards the left, the robot will start turning in place"
          n534 = Unbundle By Name(w1170) -> ("DriveRef"=w1161:T2)
          n535 = call "Custom Tank.vi"("RobotDriveDevRef 2"=w1161, "Left axis value"=-0.75 ("LeftMotorsSpeed"), "Right axis value"=0.75 ("RightMotorsSpeed")) -> ("Middle Left Motor"=w1154:T3, "Middle Right Motor"=w1153:T3)  [unwired: 8 in, 3 out]
          n536 = call <vilib>:"WPI_CANTalonSRX_SetSensorPosition.vi"("New Sensor Position"=0.0, "CAN Talon SRX Ref"=w1154) -> ("CAN Talon SRX Ref"=w1156:T3)  [unwired: 8 in, 1 out]
          n537 = call <vilib>:"WPI_CANTalonSRX_SetSensorPosition.vi"("New Sensor Position"=0.0, "CAN Talon SRX Ref"=w1153) -> ("CAN Talon SRX Ref"=w1155:T3)  [unwired: 8 in, 1 out]
          n538 = while {
            tunnel: w1156 -> [w1202]
            tunnel: w1155 -> [w1204]
            tunnel: [w1203] -> w1171
            tunnel: [w1205] -> w1172
            tunnel: w1170 -> [w1208]
            tunnel: [w1208] -> w1169
            stop <- w1214 stop-if-true
            n539 = call <vilib>:"WPI_CANTalonSRX_GetStatus.vi"("CAN Talon SRX Ref"=w1202) -> ("Talon SRX Status"=w1207:T15)  [unwired: 8 in, 2 out]
            n540 = call <vilib>:"WPI_CANTalonSRX_GetStatus.vi"("CAN Talon SRX Ref"=w1204) -> ("Talon SRX Status"=w1206:T15)  [unwired: 8 in, 2 out]
            n541 = Wait (ms)(milliseconds to wait=u32 20) -> ()  [unwired: 1 out]
            n542 = Unbundle By Name(w1207) -> ("Encoder Position"=w1203:dbl)
            n543 = Unbundle By Name(w1206) -> ("Encoder Position"=w1205:dbl)
            n544 = global read "Robot Global Data.vi" "Vision Data"() -> (w1213:T17)
            n545 = Unbundle By Name(w1213) -> ("x"=w1212:dbl)
            n546 = In Range and Coerce(upper limit=410.0, x=w1212, lower limit=390.0) -> (In Range?=w1214:bool)  [unwired: 1 out]
          }
          n547 = flat-sequence {
            tunnel: [w1218] -> w1174
            tunnel: [w1219] -> w1173
            tunnel: w1172 -> [w1219]
            tunnel: w1171 -> [w1218]
            tunnel: w1169 -> [w1217]
            tunnel: [w1217] -> w1168
            tunnel: w1174 -> [w1224]
            tunnel: w1173 -> [w1223]
            tunnel: w1168 -> [w1225]
            tunnel: [w1225] -> w1167
            tunnel: [w1224] -> w1166
            tunnel: [w1223] -> w1165
            tunnel: [w1222] -> w1164
            tunnel: [w1221] -> w1163
            frame #0 {
              w1215 = 0.0 ("LeftMotorsSpeed")
              n548 = Unbundle By Name(w1217) -> ("DriveRef"=w1216:T2)
              n549 = Wait (ms)(milliseconds to wait=u32 500) -> ()  [unwired: 1 out]
              n550 = call "Custom Tank.vi"("RobotDriveDevRef 2"=w1216, "Left axis value"=w1215, "Right axis value"=w1215) -> ()  [unwired: 8 in, 5 out]
            }
            frame #1 {
              n551 = global read "Robot Global Data.vi" "Vision Data"() -> (w1229:T17)
              n552 = Unbundle By Name(w1229) -> ("x"=w1228:dbl, "Distance"=w1221:dbl)
              n553 = In Range and Coerce(upper limit=410.0, x=w1228, lower limit=390.0) -> (In Range?=w1222:bool)  [unwired: 1 out]
            }
          }
          n554 = case shown="False" w1164 {
            tunnel: [w1183 w1201] -> _
            tunnel: w1165 -> [_ w1201]
            tunnel: w1166 -> [_ w1200]
            tunnel: [w1184 w1200] -> _
            tunnel: w1167 -> [w1182 _]
            tunnel: [w1181 w1199] -> _
            tunnel: w1163 -> [_ w1199]
            tunnel: [TRUE ("End?") TRUE ("End?")] -> w1162
            frame False {
              # "If it isn't within range then the robot will turn in place in the other direction at a slower pace until the desired pixel range is met"
              n555 = Unbundle By Name(w1182) -> ("DriveRef"=w1179:T2)
              n556 = call "Custom Tank.vi"("RobotDriveDevRef 2"=w1179, "Left axis value"=0.4 ("LeftMotorsSpeed"), "Right axis value"=-0.4 ("RightMotorsSpeed")) -> ("Middle Left Motor"=w1176:T3, "Middle Right Motor"=w1175:T3)  [unwired: 8 in, 3 out]
              n557 = while {
                tunnel: [w1188] -> w1184
                tunnel: [w1187] -> w1183
                tunnel: [w1191] -> w1181
                tunnel: w1176 -> [w1186]
                tunnel: w1175 -> [w1185]
                stop <- w1197 stop-if-true
                n558 = call <vilib>:"WPI_CANTalonSRX_GetStatus.vi"("CAN Talon SRX Ref"=w1186) -> ("Talon SRX Status"=w1190:T15)  [unwired: 8 in, 2 out]
                n559 = call <vilib>:"WPI_CANTalonSRX_GetStatus.vi"("CAN Talon SRX Ref"=w1185) -> ("Talon SRX Status"=w1189:T15)  [unwired: 8 in, 2 out]
                n560 = Wait (ms)(milliseconds to wait=u32 20) -> ()  [unwired: 1 out]
                n561 = Unbundle By Name(w1190) -> ("Encoder Position"=w1188:dbl)
                n562 = Unbundle By Name(w1189) -> ("Encoder Position"=w1187:dbl)
                n563 = global read "Robot Global Data.vi" "Vision Data"() -> (w1196:T17)
                n564 = Unbundle By Name(w1196) -> ("x"=w1195:dbl, "Distance"=w1191:dbl)
                n565 = In Range and Coerce(upper limit=405.0, x=w1195, lower limit=395.0) -> (In Range?=w1197:bool)  [unwired: 1 out]
              }
            }
            frame True {
              # "If it is within range, then the robot moves on to the shooting state"
            }
          }
          "End?" <- w1162
        }
        frame "Shoot" {
          (unwired) T16."Turn Back"
        }
        frame "Turn Back" {
          (unwired) T16."Move Back"
        }
        frame "Move Back" {
          (unwired) T16."End"
        }
        frame "End" {
          (unwired) TRUE
          (unwired) T16."End"
        }
      }
    }
    frame "Move Arms Down/Up Test" {
      n566 = flat-sequence {
        frame #0 {
          n567 = call "Zero Dart.vi"() -> ()  [unwired: 10 in, 2 out]
        }
        frame #1 {
          n568 = while {
            stop <- "stop?" stop-if-true
            n569 = call "Set Angle.vi"("Angle(degrees)"="Angle(degrees)") -> ("Pot Position"=→"Pot Position":dbl)  [unwired: 7 in, 3 out]
          }
        }
      }
    }
  }
